vi "NI-USB-8451 SPI EEPROM Programmer.vi"() -> ()   [LabVIEW 2015]
doc: "This example shows a more generalized way to use the SPI advanced API to write data. It allows the user to change the following parameters: page size, write delay, the endianness of the address bytes, and the number of bytes in an address.\n\nThe parameters will have the following effects:\n\nTarget Page Size (bytes): This places an additional constraint on the amount of bytes written. The smaller value will be used, and that number of bytes written.\nWrite Delay Between Pages (ms): This will force a mandatory delay after writing bytes to a device.\nData Address Width: This will allow the user to specify the EEPROM Data Address as either 1 or 2 bytes.\nData Address Endianness: This control will change the ordering of the bytes in the EEPROM Data Address, note that this only has an effect if there are 2 bytes in the address.\n\nFor connection information see the NI-845x Hardware and Software manual and the manual for your specific SPI device."
uses:
  <vilib>/ni845x/ni845x.llb/ni845xControl.ctl
  <vilib>/ni845x/ni845x.llb/ni845xSpiScriptControl.ctl
  <vilib>/ni845x/ni845x.llb/NI-845x SPI Script Us Delay.vi
  <vilib>/ni845x/ni845x.llb/NI-845x SPI Script Ms Delay.vi
  <vilib>/ni845x/ni845x.llb/NI-845x SPI Close Script Reference.vi
  <vilib>/LAVA/UI Tools/Dialog/Dialog/Dialog/Dialog__lava_lib_ui_tools.lvclass
  <resource>/objmgr/NI845x.rc
panel:
  in  "Verbose?":bool
  in  "Tab Control":T1(tab)
  in  "EEPROM Program Data":string[][](table)
  out "Data Bytes Written":u8[](array[numeric]) format="%x"
  out "Read Data":u8[](array[numeric]) format="%x"
  out "Hex Table":string[][](table)
  out "Bin Table":string[][](table)
  in  "EEPROM Device Type":enum16{"Microchip 93C86", "Microchip LC56BT"}(ring)=enum."Microchip LC56BT"
  in  "Device Mode":enum16{"SPI", "I2C", "DIO"}(ring)
  in  "CS Idle Level":enum16{"Low (Assert High)", "High (Assert Low)"}(ring)
  in  "CLK Phase (CPHS)":i32(ring) items=["0 (First Edge)", "1 (Second Edge)"]
  in  "CLK Polarity (CPOL)":i32(ring) items=["0 (Idle Low)", "1 (Idle High)"]
  in  "IO Level (V)":i32(ring)=33 items=["3.3V"=33, "2.5V"=25, "1.8V"=18, "1.5V"=15, "1.2V"=12]
  in  "CS/SS":u32
  in  "NI8451 Device ID":T2="NI-8451"
  in  "CLK Rate (kHz)":u16=2000
  in  "Config INI Save":bool
  in  "Help":bool
  in  "QUIT":bool
  in  "Data Width":enum16{"8 bits", "16 bits"}(ring)
  in  "Address Width":enum16{"8 bits", "16 bits"}(ring)
  in  "Bit Pattern (Write All)":T3(ring)=enum."All ONES"
  in  "Data Address Endianness":bool=TRUE
  in  "Page Write Delay (ms)":u8=3
  in  "Target Page Size (bytes)":i32=2 min=2 max=65535 step=2 format="%04x"
  in  "EEPROM Address (u8)":u16 format="%04x"
  in  "Number of Bytes (Read)":i16=256 min=4 step=4 format="%04x"
  in  "WRAL":u8=17 format="%08b"
  in  "ERAL":u8=18 format="%08b"
  in  "EWEN":u8=19 format="%08b"
  in  "READ":u8=6 format="%08b"
  in  "WRITE":u8=5 format="%08b"
  in  "EWDS":u8=16 format="%08b"
  in  "Write ALL Device":bool
  in  "Erase ALL Device":bool
  in  "Read Device":bool
  in  "Program Device":bool
  in  "SPI Script Reference":T4
  # "NI-USB-8451 SPI/I2C EEPROM Programmer\n(for 8-bit Devices Only)"
  # "NI-8451 Device Configuration"
  # "Slave Device Configur ation"
  # "Big Endian"
  # "Little Endian"
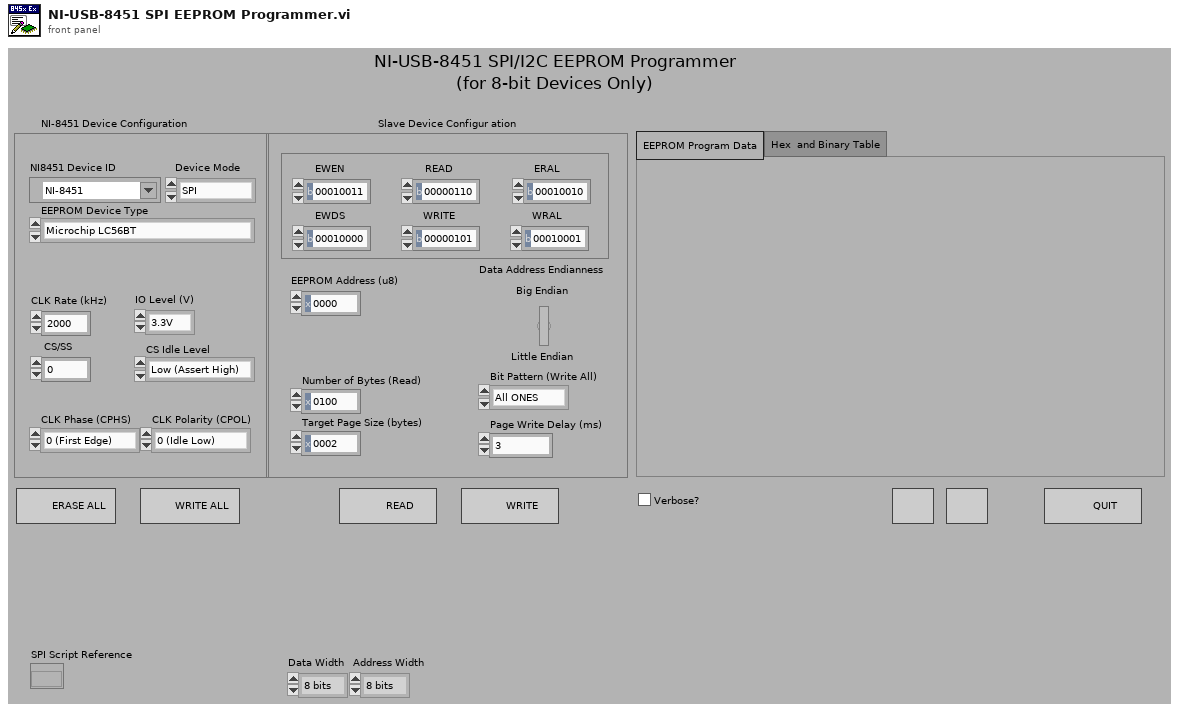
[diagram p1: front panel]
types:
  T1 = enum32{"EEPROM Program Data", "Hex  and Binary Table"}
  T2 = typedef "ni845xControl.ctl" = refnum<k21>
  T3 = enum8{"0xEE (0b11101110)", "0xAA (0b10101010)", "0x55 (0b01010101)", "All ONES", "All ZEROES", ""}
  T4 = typedef "ni845xSpiScriptControl.ctl" = refnum<k20>
  T5 = enum32{"Invalid", "Standard", "Closed", "Hidden", "Minimized", "Maximized"}
  T6 = enum32{"invalid app kind", "Development System", "Run Time System", "Student Edition", "Embedded LabVIEW", "Evaluation", "Custom"}
  T7 = cluster{"INI Path":path, "SPI Script Reference":T4, "NI8451 Device ID":T2, "Device Mode":enum16{"SPI", "I2C", "DIO"}, "EEPROM Device Type":enum16{"Microchip 93C86", "Microchip LC56BT"}, "Core":cluster{"Current VI Reference":refnum<vi>, "Close Panel on Exit?":bool}, "IO Level (V)":i32, "CS/SS":u32, "CLK Rate (kHz)":u16, "CLK Polarity (CPOL)":i32, "CLK Phase (CPHS)":i32, " Address Width":enum16{"8 bits", "16 bits"}, "Data Width":enum16{"8 bits", "16 bits"}, "EEPROM Address (u8)":u16, "Number of Bytes (Read)":i16, "Target Page Size (bytes)":i32, "Page Write Delay (ms)":u8, "Array of Write Cluster Information":cluster{"EEPROM Address":u16, "Length":u32, "Data Index":u32}[], "CS Idle Level":enum16{"Low (Assert High)", "High (Assert Low)"}, "script read index":u32, "Bit Pattern (Write All)":enum8{"0xEE (0b11101110)", "0xAA (0b10101010)", "0x55 (0b01010101)", "All ONES", "All ZEROES", ""}, "READ":u8, "WRITE":u8, "EWEN":u8, "EWDS":u8, "WRAL":u8, "ERAL":u8, "Hex Table":string[][], "Bin Table ":string[][], "EEPROM Program Data ":string[][], "Read Data":u8[], "Data Bytes Written":u8[], "Data Address Endianness":bool, "Verbose?":bool}
  T8 = cluster{"Current VI Reference":refnum<vi>, "Close Panel on Exit?":bool}
  T9 = cluster{"EEPROM Address":u16, "Length":u32, "Data Index":u32}[]
  T10 = typedef "imagedata.ctl" = cluster{"image type":i32, "image depth":i32, "image":u8[], "mask":u8[], "colors":u32[], "Rectangle":cluster{"left":i16, "top":i16, "right":i16, "bottom":i16}}
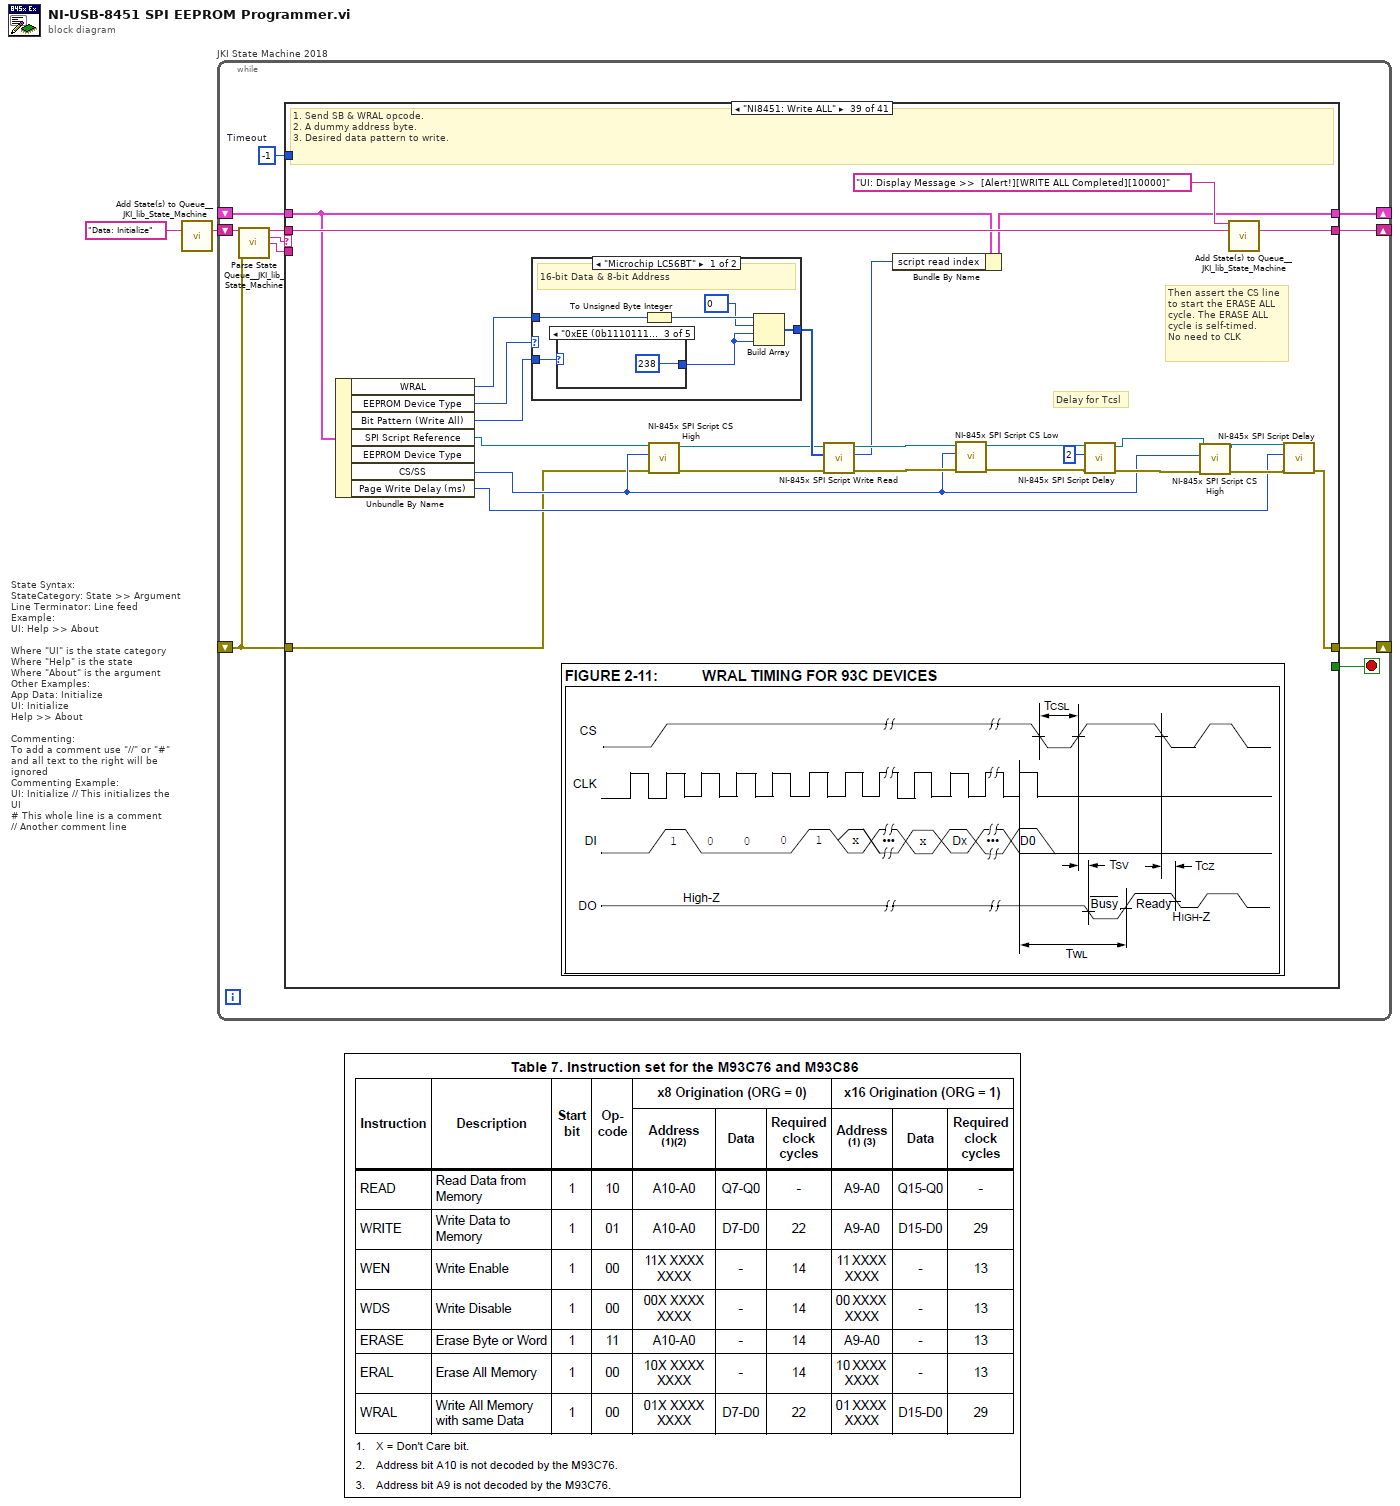
[diagram p0: block diagram]
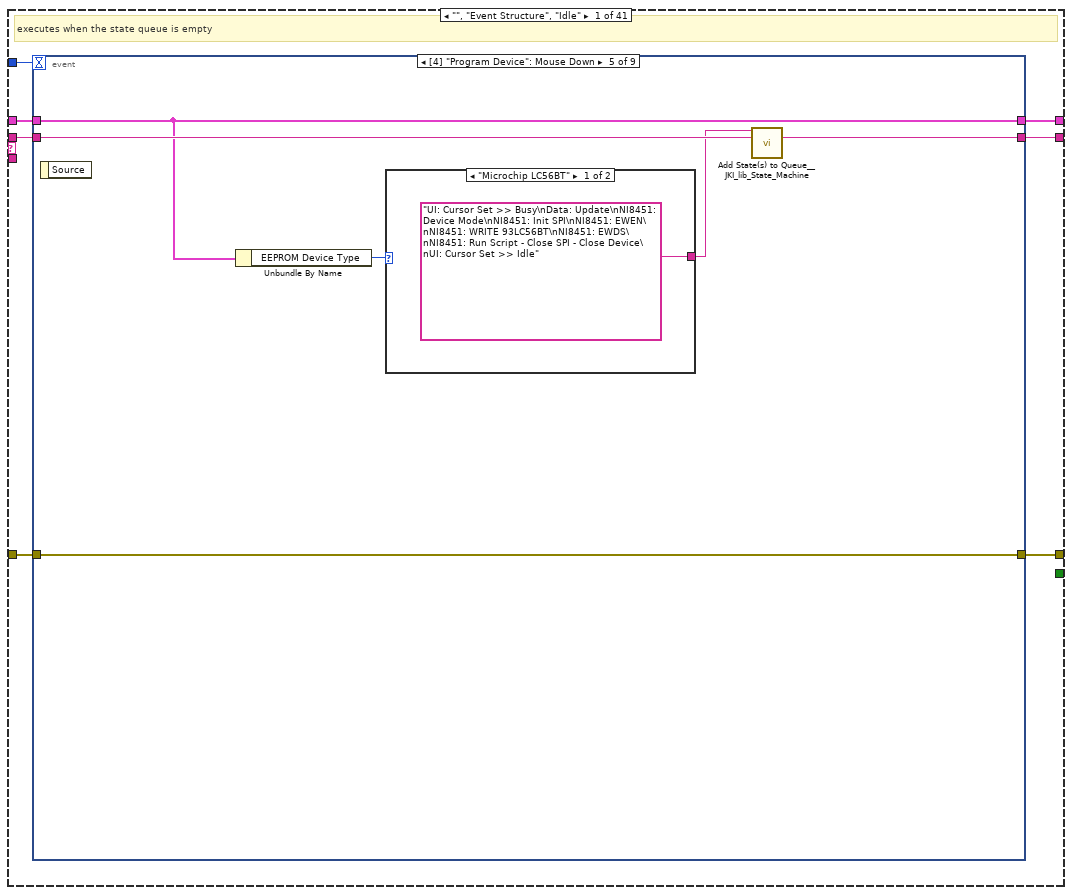
[diagram p2: hidden frame]
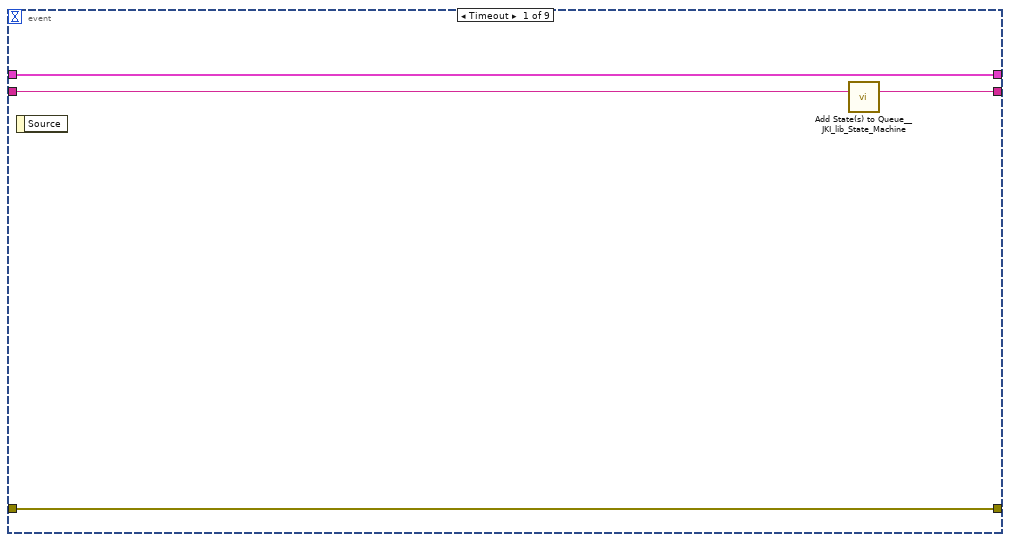
[diagram p3: hidden frame]
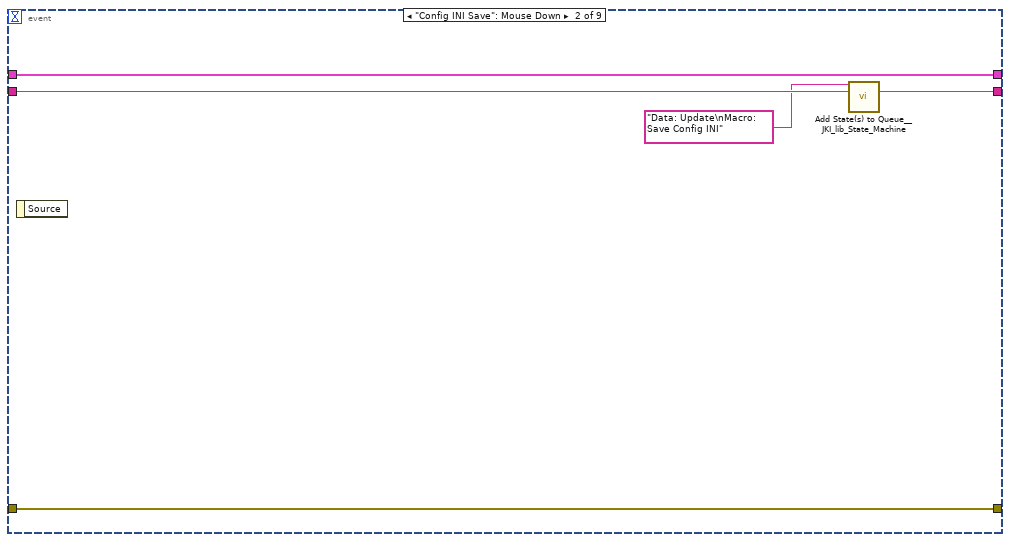
[diagram p4: hidden frame]
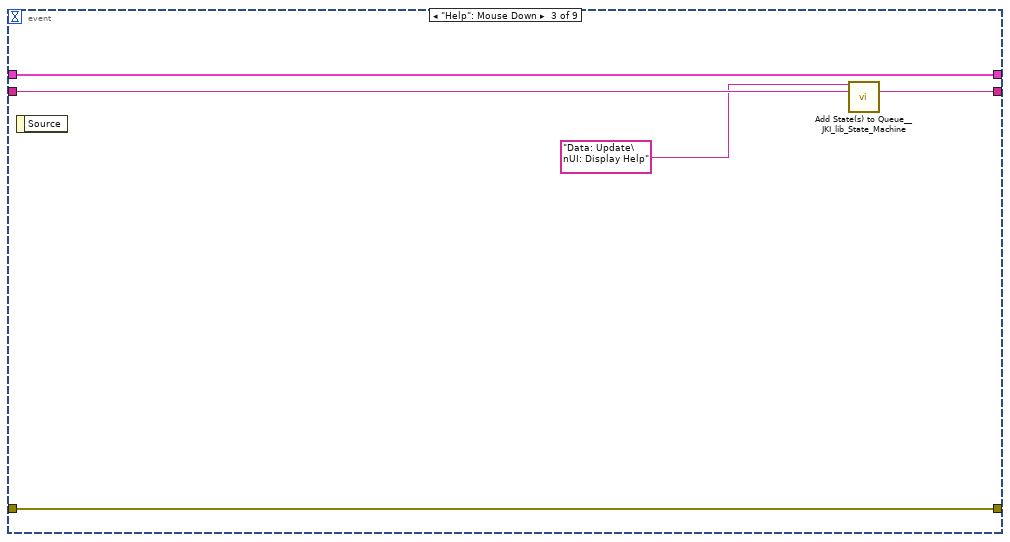
[diagram p5: hidden frame]
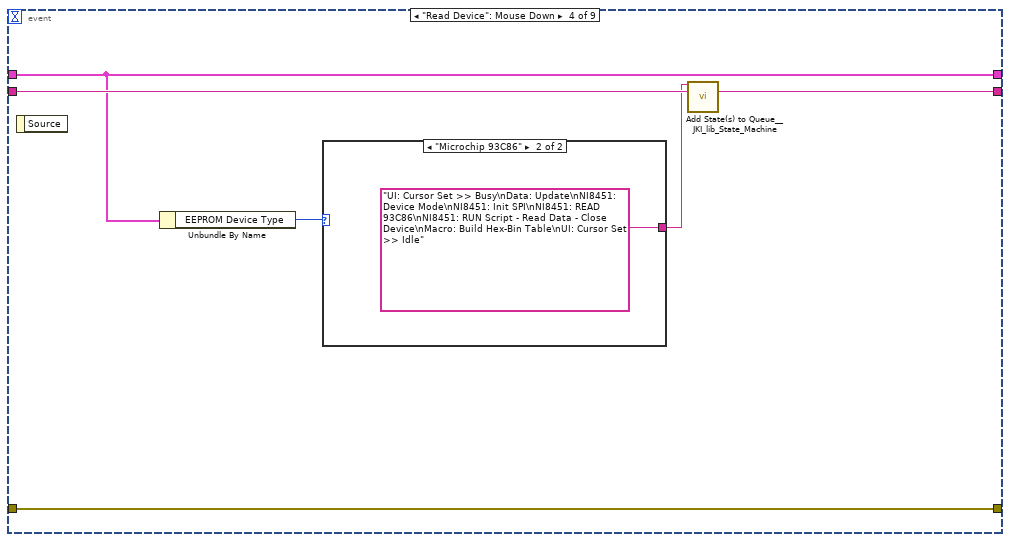
[diagram p6: hidden frame]
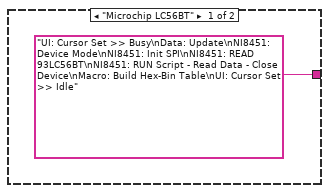
[diagram p7: hidden frame]
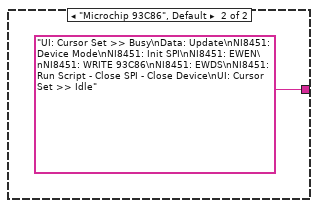
[diagram p8: hidden frame]
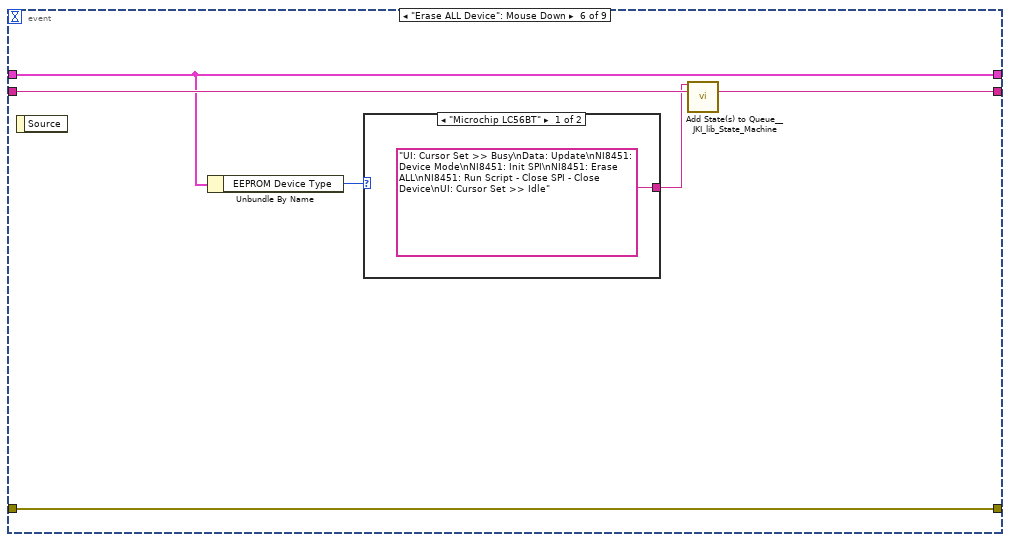
[diagram p9: hidden frame]
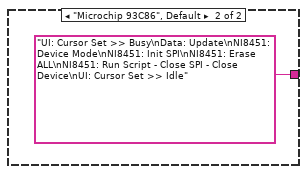
[diagram p10: hidden frame]
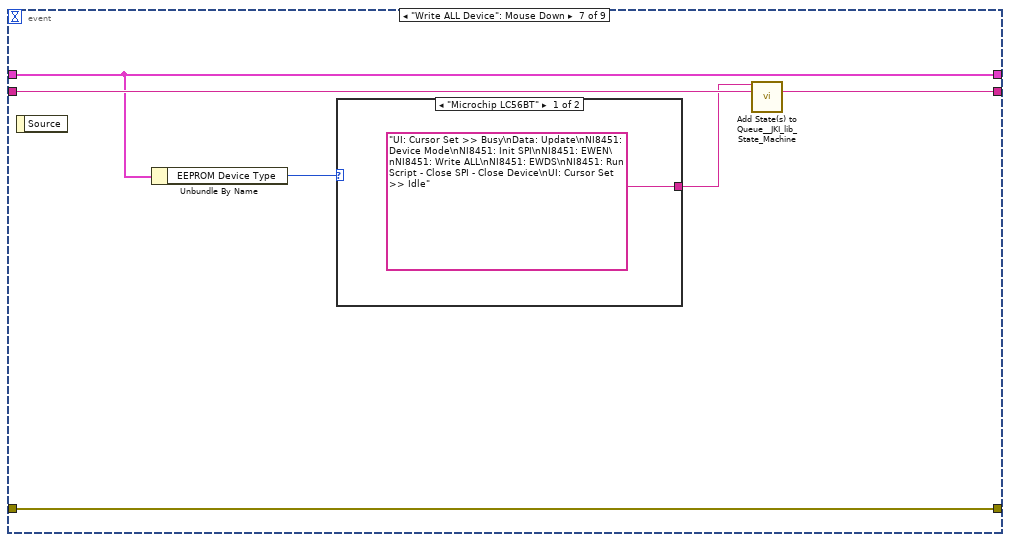
[diagram p11: hidden frame]
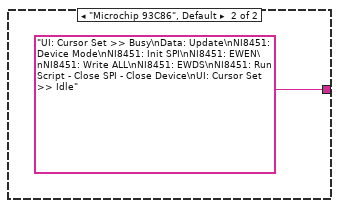
[diagram p12: hidden frame]
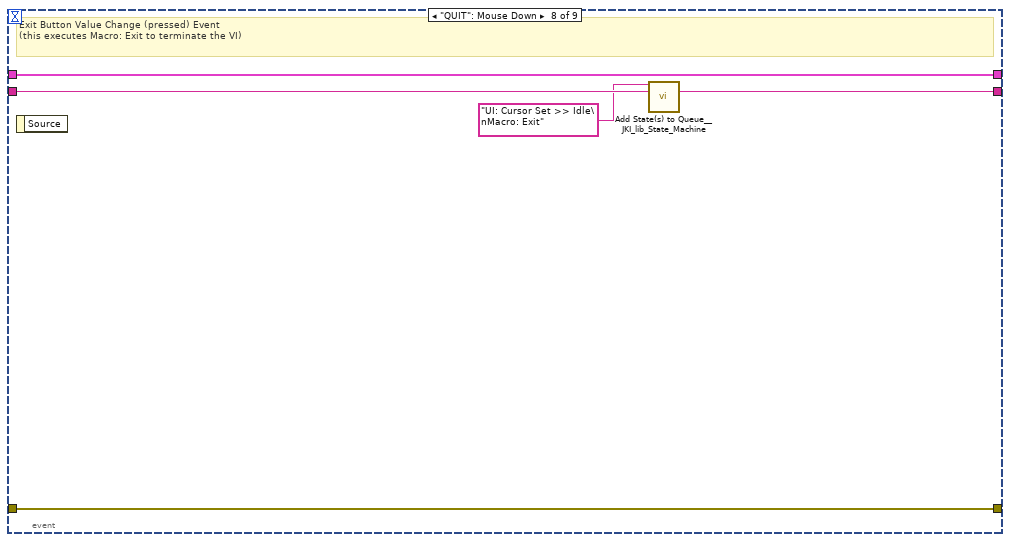
[diagram p13: hidden frame]
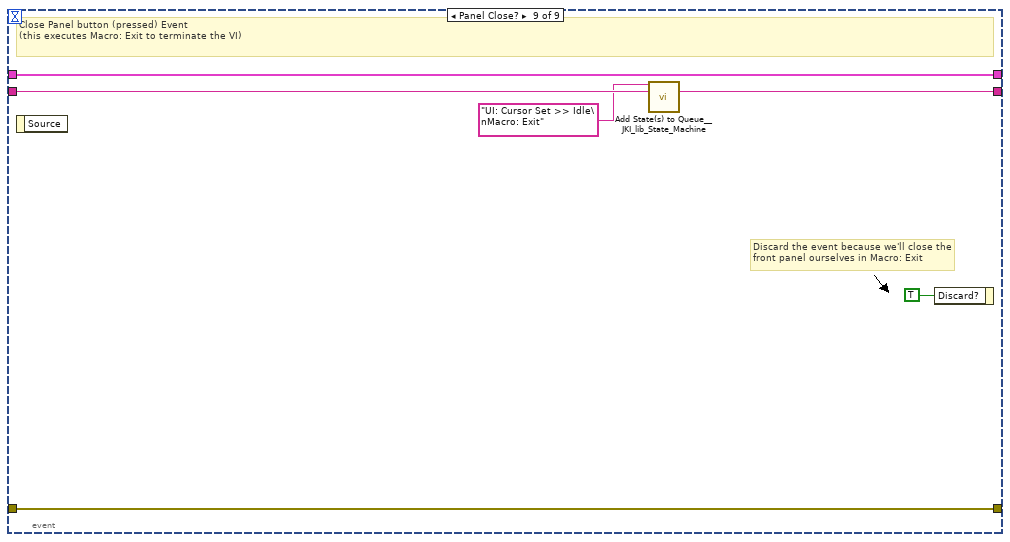
[diagram p14: hidden frame]
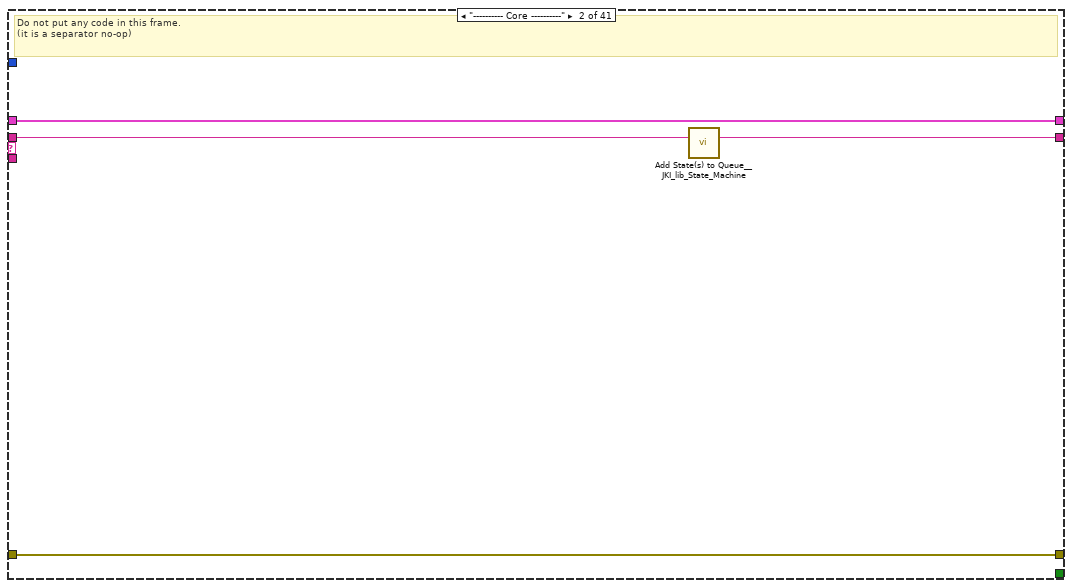
[diagram p15: hidden frame]
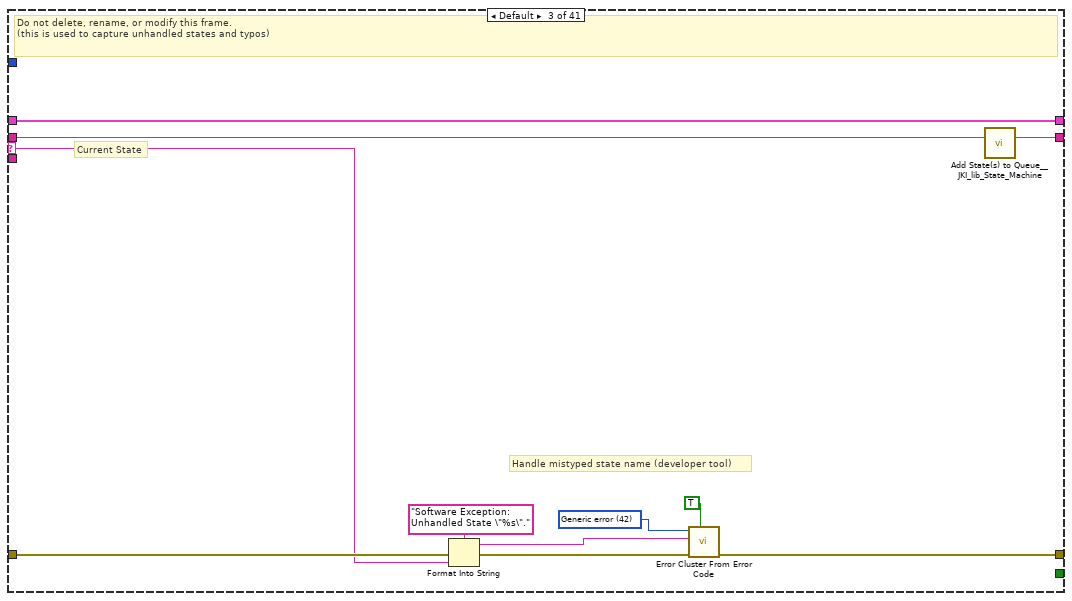
[diagram p16: hidden frame]
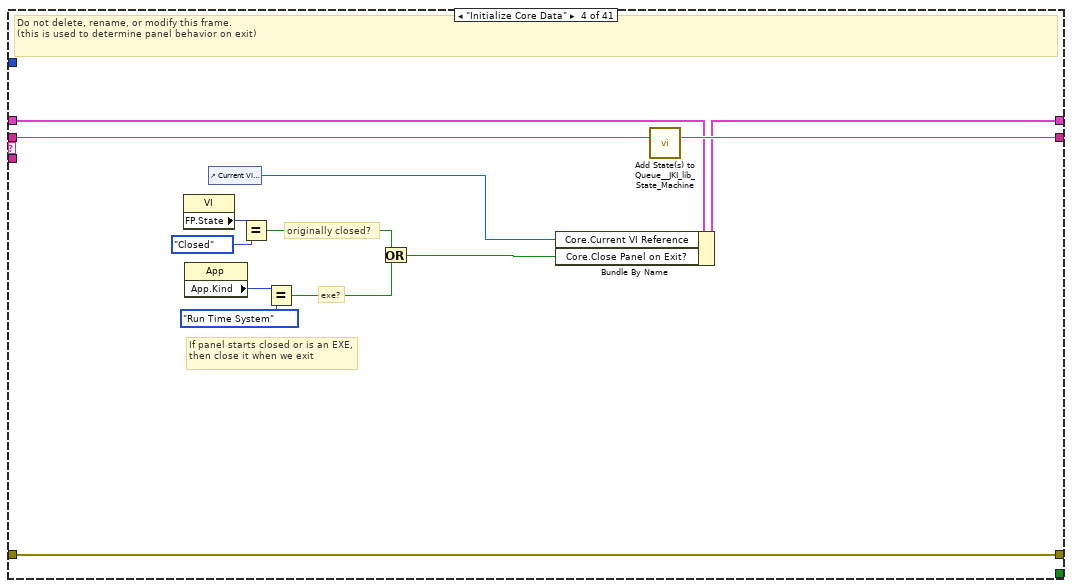
[diagram p17: hidden frame]
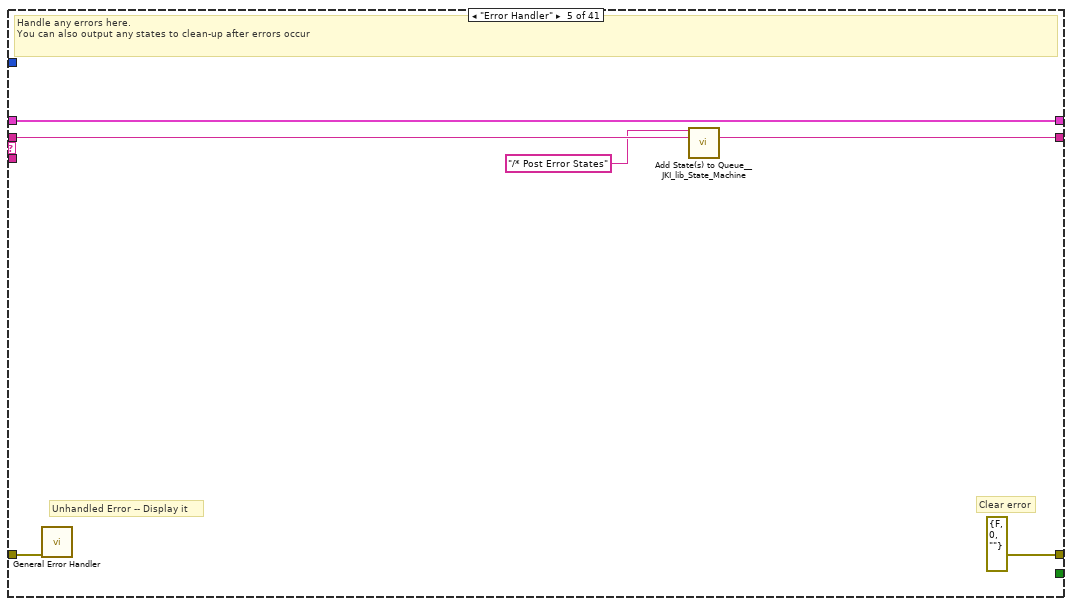
[diagram p18: hidden frame]
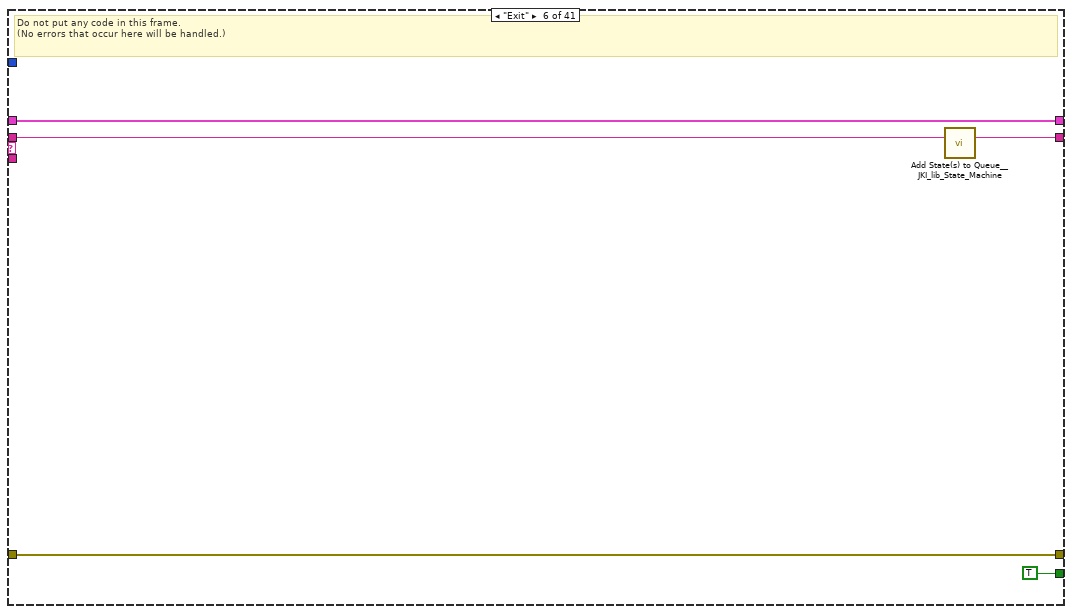
[diagram p19: hidden frame]
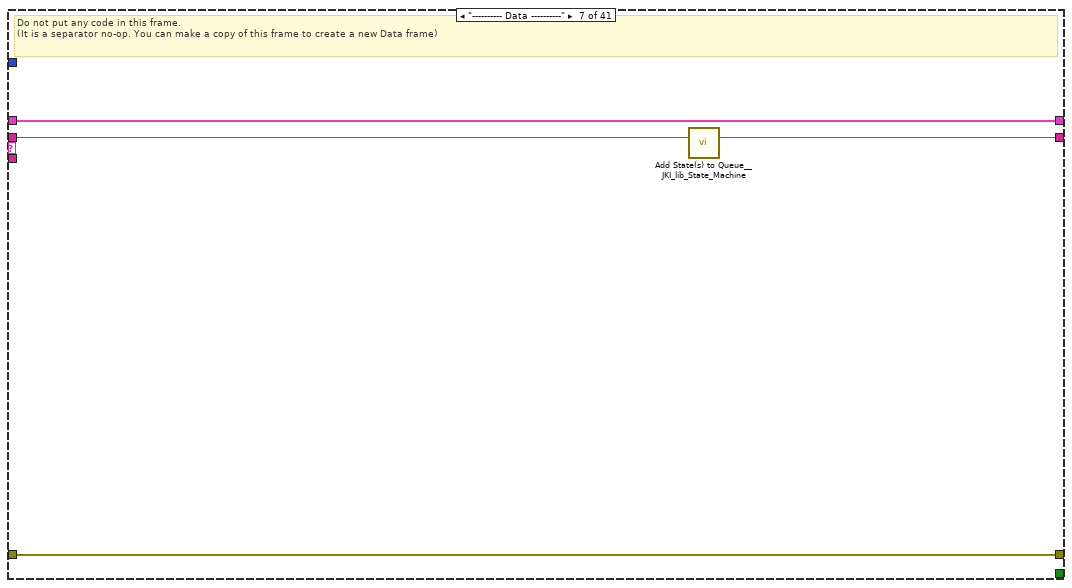
[diagram p20: hidden frame]
diagram:
  # "State Syntax:\nStateCategory: State >> Argument\nLine Terminator: Line feed\nExample:\nUI: Help >> About\n\nWhere \"UI\" is the state category\nWhere \"Help\" is the state\nWhere \"About\" is the argument\nOther Examples:\nApp Data: Initialize\nUI: Initialize\nHelp >> About\n\nCommenting:\nTo add a comment use \"//\" or \"#\" and all text to the right will be ignored\nCommenting Example:\nUI: Initialize // This initializes the UI\n# This whole line is a comment\n// Another comment line"
  n1 = call <vilib>:"Add State(s) to Queue__JKI_lib_State_Machine.vi"("State(s) in (\"\")"="Data: Initialize") -> ("States Out"=w2:string)  [unwired: 14 in]
  n2 = while "JKI State Machine 2018" {
    shift-right: [w6] -> _
    shift-left: _ -> [w5]
    shift-right: [w9] -> _
    shift-left: _ -> [w3]
    shift-right: [w8] -> _
    shift-left: w2 -> [w10]
    stop <- w7 stop-if-true
    w4 = -1  # Timeout
    n3 = call <vilib>:"Parse State Queue__JKI_lib_State_Machine.vi"("State Queue"=w10, "Error In (no error)"=w3) -> ("Remaining States"=w12:string, "Current State"=w13:string, "Arguments"=w11:string)  [unwired: 11 in]
    n4 = case shown="\"NI8451: Write ALL\"" w13 {
      selector: w13 -> [_ _ w82 _ _ _ _ _ _ _ _ _ _ _ _ _ _ _ _ _ _ _ _ _ _ _ _ _ _ _ _ _ _ _ _ _ _ _ _ _ _]
      tunnel: w12 -> [w20 w81 w86 w105 w111 w116 w120 w165 w190 w196 w200 w204 w210 w221 w296 w304 w341 w359 w369 w383 w431 w443 w455 w459 w463 w466 w470 w472 w501 w526 w577 w610 w677 w735 w805 w889 w985 w1039 w1103 w1143 w1156]
      tunnel: w11 -> [_ _ _ _ _ _ _ _ _ _ _ _ w205 w215 _ w300 _ _ _ _ _ _ _ _ _ _ _ _ _ _ _ _ _ _ _ _ _ _ _ _ _]
      tunnel: w5 -> [w18 w78 w84 w98 w108 w114 w117 _ w169 w191 w197 w202 w208 w217 w294 w298 w338 w357 w366 w380 w424 w437 w446 w456 w460 w464 w467 w474 w491 w517 w569 w607 w671 w732 w801 w886 w978 w1033 w1098 w1136 w1149]
      tunnel: [w17 w79 w88 w102 errorcluster {"status"=FALSE, "code"=0, "source"=""} ("error out") w113 w118 w130 w188 w192 w198 w201 w206 w218 w293 w302 w339 w349 w367 w381 w420 w440 w449 w457 w461 w465 w468 w475 w481 w518 w557 w601 w661 w726 w799 w879 w979 w1015 w1082 w1138 w1151] -> w9
      tunnel: w3 -> [w16 w79 w87 w102 w107 w113 w118 w125 w188 w193 w198 w201 w207 w219 w291 w301 w339 w348 w367 w381 w429 w441 w450 w457 w461 w465 w468 w475 w485 w519 w568 w608 w657 w733 w800 w887 w975 w1034 w1079 w1139 w1152]
      tunnel: [w19 w80 w85 w104 w110 w115 w119 w164 w189 w195 w199 w203 w209 w220 w295 w303 w340 w358 w368 w382 w430 w442 w454 w458 w462 w466 w469 w476 w500 w525 w576 w609 w676 w734 w804 w888 w984 w1038 w1102 w1142 w1155] -> w8
      tunnel: [_ _ _ _ _ TRUE _ _ _ _ _ _ _ _ _ _ _ _ _ _ _ _ _ _ _ _ _ _ _ _ _ _ _ _ _ _ _ _ _ _ _] -> w7
      tunnel: [w15 w78 w84 w103 w108 w114 w117 w137 w187 w191 w197 w202 w208 w217 w294 w298 w338 w357 w366 w375 w424 w437 w446 w456 w460 w464 w467 w474 w480 w517 w565 w605 w668 w730 w795 w882 w978 w1019 w1086 w1126 w1149] -> w6
      tunnel: w4 -> [w14 _ _ _ _ _ _ _ _ _ _ _ _ _ _ _ _ _ _ _ _ _ _ _ _ _ _ _ _ _ _ _ _ _ _ _ _ _ _ _ _]
      frame "", "Event Structure", "Idle" {
        # "executes when the state queue is empty"
        n5 = event shown="[4] \"Program Device\": Mouse Down" {
          selector: _ -> [_ _ _ _ _ _ _ _ _]
          dyn-events: _ -> [_ _ _ _ _ _ _ _ _]
          timeout: w14 -> [_ _ _ _ _ _ _ _ _]
          tunnel: w20 -> [w24 w29 w34 w39 w47 w55 w63 w71 w77]
          tunnel: [w23 w28 w33 w38 w46 w54 w62 w70 w76] -> w19
          tunnel: w18 -> [w21 w26 w31 w36 w44 w52 w60 w68 w74]
          tunnel: [w22 w27 w32 w40 w48 w56 w64 w69 w75] -> w17
          tunnel: w16 -> [w22 w27 w32 w40 w48 w56 w64 w69 w75]
          tunnel: [w21 w26 w31 w36 w44 w52 w60 w68 w74] -> w15
          event Timeout {
            n6 = event-data() -> ()  [unwired: 1 in, 1 out]
            n7 = call <vilib>:"Add State(s) to Queue__JKI_lib_State_Machine.vi"("State(s) in (\"\")"=w24) -> ("States Out"=w23:string)  [unwired: 14 in]
          }
          event "Config INI Save": Mouse Down {
            n8 = event-data() -> ()  [unwired: 1 in, 1 out]
            n9 = call <vilib>:"Add State(s) to Queue__JKI_lib_State_Machine.vi"("State(s) in Front (\"\")"="Data: Update\nMacro: Save Config INI" ("State(s) in Front (\"\")"), "State(s) in (\"\")"=w29) -> ("States Out"=w28:string)  [unwired: 13 in]
          }
          event "Help": Mouse Down {
            n10 = event-data() -> ()  [unwired: 1 in, 1 out]
            n11 = call <vilib>:"Add State(s) to Queue__JKI_lib_State_Machine.vi"("State(s) in Front (\"\")"="Data: Update\nUI: Display Help" ("State(s) in Front (\"\")"), "State(s) in (\"\")"=w34) -> ("States Out"=w33:string)  [unwired: 13 in]
          }
          event "Read Device": Mouse Down {
            n12 = event-data() -> ()  [unwired: 1 in, 1 out]
            n13 = Unbundle By Name(w36) -> ("EEPROM Device Type"=w35:enum16{"Microchip 93C86", "Microchip LC56BT"})
            n14 = case shown="\"Microchip 93C86\"" w35 {
              tunnel: ["UI: Cursor Set >> Busy\nData: Update\nNI8451: Device Mode\nNI8451: Init SPI\nNI8451: READ 93LC56BT\nNI8451: RUN Script - Read Data - Close Device\nMacro: Build Hex-Bin Table\nUI: Cursor Set >> Idle" ("State(s) in Front (\"\")") "UI: Cursor Set >> Busy\nData: Update\nNI8451: Device Mode\nNI8451: Init SPI\nNI8451: READ 93C86\nNI8451: RUN Script - Read Data - Close Device\nMacro: Build Hex-Bin Table\nUI: Cursor Set >> Idle" ("State(s) in Front (\"\")")] -> w37
              frame "Microchip LC56BT" {
              }
              frame "Microchip 93C86" {
              }
            }
            n15 = call <vilib>:"Add State(s) to Queue__JKI_lib_State_Machine.vi"("State(s) in Front (\"\")"=w37, "State(s) in (\"\")"=w39) -> ("States Out"=w38:string)  [unwired: 13 in]
          }
          event "Program Device": Mouse Down {
            n16 = event-data() -> ()  [unwired: 1 in, 1 out]
            n17 = Unbundle By Name(w44) -> ("EEPROM Device Type"=w43:enum16{"Microchip 93C86", "Microchip LC56BT"})
            n18 = case shown="\"Microchip LC56BT\"" w43 {
              tunnel: ["UI: Cursor Set >> Busy\nData: Update\nNI8451: Device Mode\nNI8451: Init SPI\nNI8451: EWEN\nNI8451: WRITE 93LC56BT\nNI8451: EWDS\nNI8451: Run Script - Close SPI - Close Device\nUI: Cursor Set >> Idle" ("State(s) in Front (\"\")") "UI: Cursor Set >> Busy\nData: Update\nNI8451: Device Mode\nNI8451: Init SPI\nNI8451: EWEN\nNI8451: WRITE 93C86\nNI8451: EWDS\nNI8451: Run Script - Close SPI - Close Device\nUI: Cursor Set >> Idle" ("State(s) in Front (\"\")")] -> w45
              frame "Microchip LC56BT" {
              }
              frame "Microchip 93C86", Default {
              }
            }
            n19 = call <vilib>:"Add State(s) to Queue__JKI_lib_State_Machine.vi"("State(s) in Front (\"\")"=w45, "State(s) in (\"\")"=w47) -> ("States Out"=w46:string)  [unwired: 13 in]
          }
          event "Erase ALL Device": Mouse Down {
            n20 = event-data() -> ()  [unwired: 1 in, 1 out]
            n21 = Unbundle By Name(w52) -> ("EEPROM Device Type"=w51:enum16{"Microchip 93C86", "Microchip LC56BT"})
            n22 = case shown="\"Microchip LC56BT\"" w51 {
              tunnel: ["UI: Cursor Set >> Busy\nData: Update\nNI8451: Device Mode\nNI8451: Init SPI\nNI8451: Erase ALL\nNI8451: Run Script - Close SPI - Close Device\nUI: Cursor Set >> Idle" ("State(s) in Front (\"\")") "UI: Cursor Set >> Busy\nData: Update\nNI8451: Device Mode\nNI8451: Init SPI\nNI8451: Erase ALL\nNI8451: Run Script - Close SPI - Close Device\nUI: Cursor Set >> Idle" ("State(s) in Front (\"\")")] -> w53
              frame "Microchip LC56BT" {
              }
              frame "Microchip 93C86", Default {
              }
            }
            n23 = call <vilib>:"Add State(s) to Queue__JKI_lib_State_Machine.vi"("State(s) in Front (\"\")"=w53, "State(s) in (\"\")"=w55) -> ("States Out"=w54:string)  [unwired: 13 in]
          }
          event "Write ALL Device": Mouse Down {
            n24 = event-data() -> ()  [unwired: 1 in, 1 out]
            n25 = Unbundle By Name(w60) -> ("EEPROM Device Type"=w59:enum16{"Microchip 93C86", "Microchip LC56BT"})
            n26 = case shown="\"Microchip LC56BT\"" w59 {
              tunnel: ["UI: Cursor Set >> Busy\nData: Update\nNI8451: Device Mode\nNI8451: Init SPI\nNI8451: EWEN\nNI8451: Write ALL\nNI8451: EWDS\nNI8451: Run Script - Close SPI - Close Device\nUI: Cursor Set >> Idle" ("State(s) in Front (\"\")") "UI: Cursor Set >> Busy\nData: Update\nNI8451: Device Mode\nNI8451: Init SPI\nNI8451: EWEN\nNI8451: Write ALL\nNI8451: EWDS\nNI8451: Run Script - Close SPI - Close Device\nUI: Cursor Set >> Idle" ("State(s) in Front (\"\")")] -> w61
              frame "Microchip LC56BT" {
              }
              frame "Microchip 93C86", Default {
              }
            }
            n27 = call <vilib>:"Add State(s) to Queue__JKI_lib_State_Machine.vi"("State(s) in Front (\"\")"=w61, "State(s) in (\"\")"=w63) -> ("States Out"=w62:string)  [unwired: 13 in]
          }
          event "QUIT": Mouse Down {
            # "Exit Button Value Change (pressed) Event\n(this executes Macro: Exit to terminate the VI)"
            n28 = event-data() -> ()  [unwired: 1 in, 1 out]
            n29 = call <vilib>:"Add State(s) to Queue__JKI_lib_State_Machine.vi"("State(s) in Front (\"\")"="UI: Cursor Set >> Idle\nMacro: Exit", "State(s) in (\"\")"=w71) -> ("States Out"=w70:string)  [unwired: 13 in]
          }
          event Panel Close? {
            # "Discard the event because we'll close the front panel ourselves in Macro: Exit"
            # "Close Panel button (pressed) Event\n(this executes Macro: Exit to terminate the VI)"
            n30 = event-data() -> ()  [unwired: 1 in, 1 out]
            n31 = call <vilib>:"Add State(s) to Queue__JKI_lib_State_Machine.vi"("State(s) in Front (\"\")"="UI: Cursor Set >> Idle\nMacro: Exit", "State(s) in (\"\")"=w77) -> ("States Out"=w76:string)  [unwired: 13 in]
            n32 = event-data("Discard?"=TRUE) -> ()  [unwired: 1 in, 1 out]
          }
        }
      }
      frame "---------- Core ----------" {
        # "Do not put any code in this frame.\n(it is a separator no-op)"
        n33 = call <vilib>:"Add State(s) to Queue__JKI_lib_State_Machine.vi"("State(s) in (\"\")"=w81) -> ("States Out"=w80:string)  [unwired: 14 in]
      }
      frame Default {
        w91 = 42 items=["No error", "Argument error", "Memory is full", "Out of zone", "End of file", "File already open", "Generic file I/O error", "File not found", "File permission error", "Disk is full", "Duplicate path", "Too many files open", "System feature not enabled", "Resource file not found", "Cannot add resource", "Resource not found", "Image not found", "Image memory error", "Pen does not exist", "Config type invalid", "Config token not found", "Config parse error", "Config memory error", "Bad external code format", "Bad external code offset", "External code not present", "Null window", "Destroy window error", "Null menu", "Print aborted", "Bad print record", "Print driver error", "Windows error during printing", "Memory error during printing", "Print dialog error", "Generic print error", "Invalid device refnum", "Device not found", "Device parameter error", "Device unit error", "Cannot open device", "Device call aborted", "Generic error", "Cancelled by user", "Object ID too low", "Object ID too high", "Object not in heap", "Unknown heap", "Unknown object (invalid DefProc)", "Unknown object (DefProc not in table)", "Message out of range", "Invalid (null) method", "Unknown message", "Manager call not supported", "Bad address", "Network operation in progress", "Network operation timed out", "Connection is busy", "Network attribute not supported", "Network error", "Address in use", "System out of memory", "Connection aborted", "Connection refused", "Not connected", "Already connected", "Connection closed", "Initialization error (interapplication manager)", "Bad occurrence", "Wait on unbound occurrence handler", "Occurrence queue overflow", "Datalog type conflict", "Unused", "Unrecognized type (interapplication manager)", "Memory corrupt", "Failed to make temporary DLL", "Old CIN version", "Drag socket not found", "Failed to load drop-object", "Failed to register OLE object", "Failed to release OLE object", "Format specifier type mismatch", "Unknown format specifier", "Too few format specifiers", "Too many format specifiers", "Scan failed", "Newer CIN version", "Error converting to variant", "Runtime menu error", "Password tampered", "Variant attribute not found", "Incompatible variant data type", "Event data is not available", "Event Store is not present", "Occurrence is not found", "Event Queue is not created", "Event info is not available", "Refnum passed is NULL", "Error retrieving Class GUID", "Error retrieving CoClass GUID", "Error retrieving TypeLib GUID.", "Bad built application magic bytes.", "Specific driver is different from the specific driver associated with the Logical Name.", "There is no session opened to the class driver.", "Max Error", "MAX - Error with config objects", "MAX - Error loading configuration", "MAX - Group not supported"]
        # "Current State"
        # "Handle mistyped state name (developer tool)"
        # "Do not delete, rename, or modify this frame.\n(this is used to capture unhandled states and typos)"
        n34 = Format Into String(format string="Software Exception: Unhandled State \"%s\"." ("message"), error in=w87, w82) -> (resulting string=w90:string, error out=w89:errorcluster)  [unwired: 1 in]
        n35 = call <vilib>:"Error Cluster From Error Code.vi"("show call chain? (False)"=TRUE, "error in (no error)"=w89, "error message (\"\")"=w90, "error code (0)"=w91) -> ("error out"=w88:errorcluster)  [unwired: 5 in]
        n36 = call <vilib>:"Add State(s) to Queue__JKI_lib_State_Machine.vi"("State(s) in (\"\")"=w86) -> ("States Out"=w85:string)  [unwired: 14 in]
      }
      frame "Initialize Core Data" {
        # "originally closed?"
        # "exe?"
        # "If panel starts closed or is an EXE, then close it when we exit"
        # "Do not delete, rename, or modify this frame.\n(this is used to determine panel behavior on exit)"
        n37 = property class="VI"() -> ("FP.State"=w95:T5)  [unwired: 2 in, 2 out]
        n38 = property class="App"() -> ("App.Kind"=w101:T6)  [unwired: 2 in, 2 out]
        n39 = control-ref of="Current VI Reference"() -> (w96:refnum<vi>)
        n40 = Equal?(x=w95, y=T5."Closed" ("Front Panel Window:State")) -> (x = y?=w93:bool)
        n41 = Equal?(x=w101, y=T6."Run Time System" ("Application:Kind")) -> (x = y?=w99:bool)
        n42 = Or(x=w93, y=w99) -> (x .or. y?=w97:bool)
        n43 = Bundle By Name(cluster=w98, "Core.Current VI Reference"=w96, "Core.Close Panel on Exit?"=w97) -> (w103:T7)
        n44 = call <vilib>:"Add State(s) to Queue__JKI_lib_State_Machine.vi"("State(s) in (\"\")"=w105) -> ("States Out"=w104:string)  [unwired: 14 in]
      }
      frame "Error Handler" {
        # "Unhandled Error -- Display it"
        # "Clear error"
        # "Handle any errors here.\nYou can also output any states to clean-up after errors occur"
        n45 = call <vilib>:"General Error Handler.vi"("error in (no error)"=w107) -> ()  [unwired: 10 in, 5 out]
        n46 = call <vilib>:"Add State(s) to Queue__JKI_lib_State_Machine.vi"("State(s) in Front (\"\")"="/* Post Error States", "State(s) in (\"\")"=w111) -> ("States Out"=w110:string)  [unwired: 13 in]
      }
      frame "Exit" {
        # "Do not put any code in this frame.\n(No errors that occur here will be handled.)"
        n47 = call <vilib>:"Add State(s) to Queue__JKI_lib_State_Machine.vi"("State(s) in (\"\")"=w116) -> ("States Out"=w115:string)  [unwired: 14 in]
      }
      frame "---------- Data ----------" {
        # "Do not put any code in this frame.\n(It is a separator no-op. You can make a copy of this frame to create a new Data frame)"
        n48 = call <vilib>:"Add State(s) to Queue__JKI_lib_State_Machine.vi"("State(s) in (\"\")"=w120) -> ("States Out"=w119:string)  [unwired: 14 in]
      }
      frame "Data: Initialize" {
        w121 = string[][] []  # Bin Table
        w122 = string[][] []  # Hex Table
        w124 = string[][] []  # Hex Table
        w127 = u8[] []  # Data Bytes Written
        w128 = u8[] []  # Read Data
        w138 = path ""  # INI Path
        w148 = u8[] [] ("Read Data")
        w153 = u32 0  # script read index
        w133 = T8 {"Current VI Reference"=refnum, "Close Panel on Exit?"=FALSE}  # Core
        # "do not delete - used by framework"
        # "Initialize variables & master cluster here\n(data names are defined by what you wire into the bundle function)"
        n49 = call "CreateWriteCluster.vi"("Page Size in Bytes"="Target Page Size (bytes)", "EEPROM Starting Address"="EEPROM Address (u8)", "Number of Bytes to Write"="Number of Bytes (Read)") -> ("Array of Write Cluster Information"=w141:T9)  [unwired: 1 in]
        n50 = control-ref of="This VI"() -> (w131:refnum<vi>)
        n51 = call "Set Config INI PATH.vi"("error in (no error)"=w125, "reference"=w131) -> ("error out"=w130:errorcluster, "appended path"=w129:path)  [unwired: 2 in]
        n52 = Bundle("INI Path"=w138, "SPI Script Reference"="SPI Script Reference", "NI8451 Device ID"="NI8451 Device ID", "Device Mode"="Device Mode", "EEPROM Device Type"="EEPROM Device Type", "Core"=w133, "IO Level (V)"="IO Level (V)", "CS/SS"="CS/SS", "CLK Rate (kHz)"="CLK Rate (kHz)", "CLK Polarity (CPOL)"="CLK Polarity (CPOL)", "CLK Phase (CPHS)"="CLK Phase (CPHS)", "Address Width"="Address Width", "Data Width"="Data Width", "EEPROM Address (u8)"="EEPROM Address (u8)", "Number of Bytes (Read)"="Number of Bytes (Read)", "Target Page Size (bytes)"="Target Page Size (bytes)", "Page Write Delay (ms)"="Page Write Delay (ms)", "Array of Write Cluster Information"=w141, "CS Idle Level"="CS Idle Level", "script read index"=w153, "Bit Pattern (Write All)"="Bit Pattern (Write All)", "READ"="READ", "WRITE"="WRITE", "EWEN"="EWEN", "EWDS"="EWDS", "WRAL"="WRAL", "ERAL"="ERAL", "Hex Table"=w122, "Bin Table"=w121, "EEPROM Program Data"="EEPROM Program Data", "Read Data"=w128, "Data Bytes Written"=w127, "Data Address Endianness"="Data Address Endianness", "Verbose?"="Verbose?") -> (w163:T7)  [unwired: 1 in]
        n53 = Bundle By Name(cluster=w163, "INI Path"=w129) -> (w137:T7)
        n54 = call <vilib>:"Add State(s) to Queue__JKI_lib_State_Machine.vi"("State(s) in Front (\"\")"="Initialize Core Data\nMacro: Initialize", "State(s) in (\"\")"=w165) -> ("States Out"=w164:string)  [unwired: 13 in]
        "Read Data" <- w148
        "Data Bytes Written" <- w148
        "Hex Table" <- w124
        "Bin Table" <- w124
      }
      frame "Data: Update" {
        # "Update the master cluster for any config changes"
        n55 = Unbundle By Name(w169) -> ("Hex Table"=w168:string[][], "Bin Table"=w167:string[][])
        n56 = local write "Hex Table"(w168) -> ()
        n57 = local write "Bin Table"(w167) -> ()
        n58 = local read "Number of Bytes (Read)"() -> (w182:i16)
        n59 = local read "Data Address Endianness"() -> (w171:bool)
        n60 = local read "Target Page Size (bytes)"() -> (w180:i32)
        n61 = local read "EEPROM Program Data"() -> (w166:string[][])
        n62 = local read "Page Write Delay (ms)"() -> (w186:u8)
        n63 = local read "EEPROM Address (u8)"() -> (w181:u16)
        n64 = local read "EEPROM Device Type"() -> (w172:enum16{"Microchip 93C86", "Microchip LC56BT"})
        n65 = local read "NI8451 Device ID"() -> (w175:T2)
        n66 = local read "Bit Pattern (Write All)"() -> (w179:T3)
        n67 = local read "Address Width"() -> (w184:enum16{"8 bits", "16 bits"})
        n68 = local read "CLK Rate (kHz)"() -> (w178:u16)
        n69 = local read "Device Mode"() -> (w174:enum16{"SPI", "I2C", "DIO"})
        n70 = local read "CS Idle Level"() -> (w185:enum16{"Low (Assert High)", "High (Assert Low)"})
        n71 = local read "IO Level (V)"() -> (w176:i32)
        n72 = local read "Data Width"() -> (w173:enum16{"8 bits", "16 bits"})
        n73 = local read "Verbose?"() -> (w170:bool)
        n74 = local read "CS/SS"() -> (w177:u32)
        n75 = call "CreateWriteCluster.vi"("Page Size in Bytes"=w180, "EEPROM Starting Address"=w181, "Number of Bytes to Write"=w182) -> ("Array of Write Cluster Information"=w183:T9)  [unwired: 1 in]
        n76 = Bundle By Name(cluster=w169, "EEPROM Device Type"=w172, "NI8451 Device ID"=w175, "Device Mode"=w174, "IO Level (V)"=w176, "CS/SS"=w177, "CLK Rate (kHz)"=w178, "Bit Pattern (Write All)"=w179, "Number of Bytes (Read)"=w182, "Target Page Size (bytes)"=w180, "Page Write Delay (ms)"=w186, "CS Idle Level"=w185, "script read index"=w184, "Data Width"=w173, "EEPROM Address (u8)"=w181, "Array of Write Cluster Information"=w183, "Data Address Endianness"=w171, "Verbose?"=w170, "EEPROM Program Data"=w166) -> (w187:T7)
        n77 = call <vilib>:"Add State(s) to Queue__JKI_lib_State_Machine.vi"("State(s) in (\"\")"=w190) -> ("States Out"=w189:string)  [unwired: 14 in]
      }
      frame "Data: Cleanup" {
        # "Cleanup any data and references, here.\n(this is called automatically, by the Macro: Exit)"
        n78 = Unbundle By Name(w191) -> ("Core.Current VI Reference"=w194:refnum<vi>)
        n79 = Close Reference(reference=w194, error in (no error)=w193) -> (error out=w192:errorcluster)
        n80 = call <vilib>:"Add State(s) to Queue__JKI_lib_State_Machine.vi"("State(s) in (\"\")"=w196) -> ("States Out"=w195:string)  [unwired: 14 in]
      }
      frame "---------- UI ----------" {
        # "Do not put any code in this frame.\n(It is a separator no-op. You can make a copy of this frame to create a new UI frame)"
        n81 = call <vilib>:"Add State(s) to Queue__JKI_lib_State_Machine.vi"("State(s) in (\"\")"=w200) -> ("States Out"=w199:string)  [unwired: 14 in]
      }
      frame "UI: Initialize" {
        # "Initialize the User Interface, here.\n(this is called automatically, by the Macro: Init)"
        n82 = call <vilib>:"Add State(s) to Queue__JKI_lib_State_Machine.vi"("State(s) in (\"\")"=w204) -> ("States Out"=w203:string)  [unwired: 14 in]
      }
      frame "UI: Cursor Set" {
        # "Argument"
        # "Set and Unset Cursor Busy.\n(Usage: \"UI: Cursor Set >> Busy|Idle\")"
        n83 = case shown="\"Busy\"" w205 {
          tunnel: w207 -> [w212 w214]
          tunnel: [w211 w213] -> w206
          frame "Idle", Default {
            n84 = call <vilib>:"Unset Busy.vi"("error in (no error)"=w212) -> ("error out"=w211:errorcluster)  [unwired: 10 in]
          }
          frame "Busy" {
            n85 = call <vilib>:"Set Busy.vi"("error in (no error)"=w214) -> ("error out"=w213:errorcluster)  [unwired: 9 in, 1 out]
          }
        }
        n86 = call <vilib>:"Add State(s) to Queue__JKI_lib_State_Machine.vi"("State(s) in (\"\")"=w210) -> ("States Out"=w209:string)  [unwired: 14 in]
      }
      frame "UI: Front Panel State" {
        # "Argument"
        # "Set Front Panel Open or Closed\n(Usage: \"UI: Front Panel State >> Open|Close\")"
        n87 = Unbundle By Name(w217) -> ("Core.Current VI Reference"=w216:refnum<vi>)
        n88 = case shown="\"Minimize\", \"Minimized\"" w215 {
          tunnel: w219 -> [w227 w242 w253 w266 w279]
          tunnel: [w229 w243 w255 w268 w281] -> w218
          tunnel: w216 -> [w228 w240 w254 w267 w280]
          frame "Open", "Standard", Default {
            w222 = T5."Standard" ("State")
            n89 = property class="VI"(reference=w228, error in=w227) -> (reference out=w225:refnum<vi>, error out=w226:errorcluster, "FP.State"=w224:T5)
            n90 = Not Equal?(x=w224, y=w222) -> (x != y?=w223:bool)
            n91 = case shown="True" w223 {
              tunnel: [w233 w235] -> w229
              tunnel: w226 -> [w232 w235]
              tunnel: w225 -> [w231 _]
              tunnel: w222 -> [w230 _]
              frame True {
                n92 = invoke class="VI" method="FP.Open"(reference=w231, error in=w232, "Activate"=TRUE, "State"=w230) -> (error out=w233:errorcluster)  [unwired: 1 in, 4 out]
              }
              frame False {
              }
            }
          }
          frame "Close", "Closed" {
            n93 = property class="VI"(reference=w240, error in=w242) -> (reference out=w239:refnum<vi>, error out=w241:errorcluster, "FP.State"=w237:T5)
            n94 = Not Equal?(x=w237, y=T5."Closed" ("Front Panel Window:State")) -> (x != y?=w236:bool)
            n95 = case shown="True" w236 {
              tunnel: [w244 w247] -> w243
              tunnel: w241 -> [w244 w246]
              tunnel: w239 -> [_ w245]
              frame False {
              }
              frame True {
                n96 = invoke class="VI" method="FP.Close"(reference=w245, error in=w246) -> (error out=w247:errorcluster)  [unwired: 1 in, 2 out]
              }
            }
          }
          frame "Hidden", "Hide" {
            w248 = T5."Hidden" ("State")
            n97 = property class="VI"(reference=w254, error in=w253) -> (reference out=w251:refnum<vi>, error out=w252:errorcluster, "FP.State"=w250:T5)
            n98 = Not Equal?(x=w250, y=w248) -> (x != y?=w249:bool)
            n99 = case shown="True" w249 {
              tunnel: [w259 w260] -> w255
              tunnel: w252 -> [w258 w260]
              tunnel: w251 -> [w257 _]
              tunnel: w248 -> [w256 _]
              frame True {
                n100 = invoke class="VI" method="FP.Open"(reference=w257, error in=w258, "State"=w256) -> (error out=w259:errorcluster)  [unwired: 2 in, 4 out]
              }
              frame False {
              }
            }
          }
          frame "Minimize", "Minimized" {
            w261 = T5."Minimized" ("State")
            n101 = property class="VI"(reference=w267, error in=w266) -> (reference out=w264:refnum<vi>, error out=w265:errorcluster, "FP.State"=w263:T5)
            n102 = Not Equal?(x=w263, y=w261) -> (x != y?=w262:bool)
            n103 = case shown="True" w262 {
              tunnel: [w272 w273] -> w268
              tunnel: w265 -> [w271 w273]
              tunnel: w264 -> [w270 _]
              tunnel: w261 -> [w269 _]
              frame True {
                n104 = invoke class="VI" method="FP.Open"(reference=w270, error in=w271, "State"=w269) -> (error out=w272:errorcluster)  [unwired: 2 in, 4 out]
              }
              frame False {
              }
            }
          }
          frame "Maximize", "Maximized" {
            w274 = T5."Maximized" ("State")
            n105 = property class="VI"(reference=w280, error in=w279) -> (reference out=w277:refnum<vi>, error out=w278:errorcluster, "FP.State"=w276:T5)
            n106 = Not Equal?(x=w276, y=w274) -> (x != y?=w275:bool)
            n107 = case shown="True" w275 {
              tunnel: [w285 w286] -> w281
              tunnel: w278 -> [w284 w286]
              tunnel: w277 -> [w283 _]
              tunnel: w274 -> [w282 _]
              frame True {
                n108 = invoke class="VI" method="FP.Open"(reference=w283, error in=w284, "State"=w282) -> (error out=w285:errorcluster)  [unwired: 2 in, 4 out]
              }
              frame False {
              }
            }
          }
        }
        n109 = call <vilib>:"Add State(s) to Queue__JKI_lib_State_Machine.vi"("State(s) in (\"\")"=w221) -> ("States Out"=w220:string)  [unwired: 14 in]
      }
      frame "UI: Display Help" {
        n110 = call <vilib>:"Read JPEG File.vi"("error in (no error)"=w291, "path to JPEG file"=path "C:/projects/AldrinA_Test_Apps/NI-845x I2C-SPI Programmer GUI/NI8451_J6_wiring.jpg" ("Path")) -> ("error out"=w290:errorcluster, "image data"=w289:T10)  [unwired: 7 in, 1 out]
        n111 = call <vilib>:"Draw Flattened Pixmap.vi"("image data"=w289, "picture"=picture data[5B]) -> ("new picture"=w288:picture)  [unwired: 7 in]
        n112 = call "Picture Prompt.vi"("error in (no error)"=w290, "2D Picture 2"=w288) -> ("error out"=w293:errorcluster)  [unwired: 9 in]
        n113 = call <vilib>:"Add State(s) to Queue__JKI_lib_State_Machine.vi"("State(s) in (\"\")"=w296) -> ("States Out"=w295:string)  [unwired: 14 in]
      }
      frame "UI: Display Message" {
        # "// Command Format:  \"UI: Display Message >> [Window Title] [Message] [Timeout]\""
        n114 = call <vilib>:"Trim Whitespace.vi"("string"=w300) -> ("trimmed string"=w299:string)  [unwired: 1 in]
        n115 = Unbundle By Name(w298) -> ("Verbose?"=w297:bool)
        n116 = case shown="True" w297 {
          tunnel: [w305 w314] -> w302
          tunnel: w301 -> [w305 w313]
          tunnel: w299 -> [_ w312]
          frame False {
          }
          frame True {
            n117 = Empty String/Path?(string/path=w312) -> (empty?=w306:bool)
            n118 = case shown="False" w306 {
              tunnel: w312 -> [w325 _]
              tunnel: [w322 w326] -> w309
              tunnel: [w321 w326] -> w308
              tunnel: [w315 -1] -> w307
              frame False {
                w318 = string[] ["[", "]"] ("delimiters (\\s,\\t,\\r,\\n)")
                n119 = Scan String For Tokens(6:w318, 9:w325) -> (1:w322:string, 2:w324:i32, 3:w323:string)  [unwired: 4 in, 1 out]
                n120 = Scan String For Tokens(6:w318, 8:w324, 9:w323) -> (1:w321:string, 2:w319:i32, 3:w320:string)  [unwired: 3 in, 1 out]
                n121 = Scan String For Tokens(6:w318, 8:w319, 9:w320) -> (1:w317:string)  [unwired: 3 in, 3 out]
                n122 = Decimal String To Number(string=w317, default (0L)=10000 ("Timeout (-1)")) -> (number=w315:i32)  [unwired: 1 in, 1 out]
              }
              frame True {
                w326 = "Important Message" ("token string")
              }
            }
            n123 = call <vilib>:"Init Dialog__lava_lib_ui_tools.vi"("error in (no error)"=w313, "Timeout (-1)"=w307, "Message"=w308, "Dialog Title"=w309) -> ("error out"=w310:errorcluster, "Dialog out"=w311:refnum<class "Dialog__lava_lib_ui_tools.lvclass">)  [unwired: 6 in]
            n124 = while {
              tunnel: w311 -> [w335]
              shift-right: [w333] -> w314
              shift-left: w310 -> [w334]
              stop <- w330 stop-if-true
              n125 = call-dynamic "Dialog Box__lava_lib_ui_tools.vi"("error in (no error)"=w334, "Dialog in"=w335) -> ("error out"=w333:errorcluster, "timed out?"=w329:bool, "Selection"=w332:string)  [unwired: 6 in, 1 out]
              n126 = case shown="\"False\", Default" w332 {
                tunnel: [TRUE FALSE] -> w331
                frame "False", Default {
                }
                frame "True" {
                }
              }
              n127 = Or(x=w331, y=w329) -> (x .or. y?=w330:bool)
              n128 = Wait (ms)(milliseconds to wait=u32 100) -> ()  [unwired: 1 out]
            }
          }
        }
        n129 = call <vilib>:"Add State(s) to Queue__JKI_lib_State_Machine.vi"("State(s) in (\"\")"=w304) -> ("States Out"=w303:string)  [unwired: 14 in]
      }
      frame "---------- Macro ----------" {
        # "Do not put any code in this frame.\n(It is a separator no-op. You can make a copy of this frame to create a new Macro frame)"
        n130 = call <vilib>:"Add State(s) to Queue__JKI_lib_State_Machine.vi"("State(s) in (\"\")"=w341) -> ("States Out"=w340:string)  [unwired: 14 in]
      }
      frame "Macro: Initialize" {
        w342 = string[][] [] ("Hex Table")
        w344 = string[] ["Address", "1", "2", "3", "4"] ("Column Header Strings[]")
        w350 = FALSE ("QUIT")
        w356 = "UI: Initialize\nUI: Front Panel State >> Open\nMacro: Load Config INI\nData: Update"  # UI: Initialize UI: Front Panel State >> Open Macro: Load Config INI Data: Update
        # "Initialization Macro\n(This is called once, when the VI starts)"
        n131 = property on="Hex Table" class="Tbl (strict)"(error in=w348, "Column Headers[]"=w344, "Number of Columns"=u32 5, "Value"=w342) -> (error out=w346:errorcluster)  [unwired: 1 in, 1 out]
        n132 = property on="Bin Table" class="Tbl (strict)"(error in=w346, "Column Headers[]"=w344, "Number of Columns"=u32 5, "Value"=w342) -> (error out=w345:errorcluster)  [unwired: 1 in, 1 out]
        n133 = property on="QUIT" class="Bool (strict)"(error in=w345, "Value"=w350) -> (error out=w352:errorcluster)  [unwired: 1 in, 1 out]
        n134 = property on="Read Device" class="Bool (strict)"(error in=w352, "Value"=w350) -> (error out=w353:errorcluster)  [unwired: 1 in, 1 out]
        n135 = property on="Program Device" class="Bool (strict)"(error in=w353, "Value"=w350) -> (error out=w354:errorcluster)  [unwired: 1 in, 1 out]
        n136 = property on="Write ALL Device" class="Bool (strict)"(error in=w354, "Value"=w350) -> (error out=w355:errorcluster)  [unwired: 1 in, 1 out]
        n137 = property on="Erase ALL Device" class="Bool (strict)"(error in=w355, "Value"=w350) -> (error out=w351:errorcluster)  [unwired: 1 in, 1 out]
        n138 = property on="Help" class="Bool (strict)"(error in=w351, "Value"=w350) -> (error out=w349:errorcluster)  [unwired: 1 in, 1 out]
        n139 = call <vilib>:"Add State(s) to Queue__JKI_lib_State_Machine.vi"("State(s) in Front (\"\")"=w356, "State(s) in (\"\")"=w359) -> ("States Out"=w358:string)  [unwired: 13 in]
      }
      frame "Macro: Exit" {
        # "Exit Macro\n(This is called once, when the VI exits)"
        n140 = Unbundle By Name(w366) -> ("Core.Close Panel on Exit?"=w365:bool)
        n141 = Select(t="UI: Front Panel State >> Close", s=w365, f="") -> (s? t:f=w362:string)
        n142 = call <vilib>:"Add State(s) to Queue__JKI_lib_State_Machine.vi"("State(s) in (\"\")"=w362, "State(s) at Back (\"\")"="Data: Cleanup\nMacro: Save Config INI\nExit") -> ("States Out"=w360:string)  [unwired: 13 in]
        n143 = call <vilib>:"Add State(s) to Queue__JKI_lib_State_Machine.vi"("State(s) in Front (\"\")"=w360, "State(s) in (\"\")"=w369) -> ("States Out"=w368:string)  [unwired: 13 in]
      }
      frame "Macro: Build Hex-Bin Table" {
        w376 = string[][] [] ("array")
        # "Update the Hex strings display post data capture from device"
        n144 = Unbundle By Name(w380) -> ("Read Data"=w379:u8[], "Target Page Size (bytes)"=w370:i32)
        n145 = Array Size(array=w379) -> (size(s)=w378:i32)
        n146 = Quotient & Remainder(x=w378, y=w370) -> (floor(x/y)=w377:i32)  [unwired: 1 out]
        n147 = Increment(x=w377) -> (x+1=w371:i32)
        n148 = for {
          N: w371 -> [_]
          shift-right: [w403] -> _
          shift-left: w379 -> [w402]
          shift-right: [w400] -> w373
          shift-left: w376 -> [w399]
          shift-right: [w391] -> w374
          shift-left: w376 -> [w390]
          tunnel: w370 -> [w386]
          i -> [w384]
          # "Extract n bytes at a time (per page size)\nRemaining elements to shift register"
          n149 = Delete From Array(array=w402, length=w386, index=0) -> (deleted portion=w404:u8[], array with subset deleted=w403:u8[])
          n150 = for {
            tunnel: w404 -> [w419] mode=indexing
            shift-right: [w417] -> _
            shift-left: "" -> [w416]
            shift-right: [w415] -> _
            shift-left: _ -> [w414]
            shift-right: [w411] -> w398
            shift-left: string[] [] ("array") -> [w409]
            shift-right: [w405] -> w393
            shift-left: _ -> [w406]
            i -> [w408]
            w412 = "\t"
            n151 = Number To Hexadecimal String(2:w419) -> (0:w418:string)  [unwired: 1 in]
            n152 = call "Hex_String_to_Binary_String.vi"("bitness"=enum16{"8", "16", "32", "64"}."8", "Hexadecimal String"=w418) -> ("Hex String"=w410:string, "Binary String"=w407:string)  [unwired: 1 in, 1 out]
            n153 = Concatenate Strings(w416, w407, w412) -> (w417:string)
            n154 = Insert Into Array(array=w406, index=w408, new element=w407) -> (w405:string[])
            n155 = Concatenate Strings(w414, w410, w412) -> (w415:string)
            n156 = Insert Into Array(array=w409, index=w408, new element=w410) -> (w411:string[])
          }
          n157 = Number To Hexadecimal String(1:i16 4 ("width (-)"), 2:w384) -> (0:w394:string)
          n158 = Increment(x=w386) -> (x+1=w385:i32)
          n159 = Build Array (concatenate)(w394, w398) -> (w397:string[])
          n160 = Build Array (concatenate)(w394, w393) -> (w395:string[])
          n161 = Reshape Array(w397, w385) -> (w396:string[])
          n162 = Reshape Array(w395, w385) -> (w392:string[])
          n163 = Insert Into Array(array=w390, index (row)=w384, new element=w392) -> (w391:string[][])  [unwired: 1 in]
          n164 = Insert Into Array(array=w399, index (row)=w384, new element=w396) -> (w400:string[][])  [unwired: 1 in]
        }
        n165 = local write "Bin Table"(w374) -> ()
        n166 = local write "Hex Table"(w373) -> ()
        n167 = call <vilib>:"Add State(s) to Queue__JKI_lib_State_Machine.vi"("State(s) in Front (\"\")"="UI: Display Message >>  [Alert!][Hex & Binary Table Parsed][10000]" ("State(s) in Front (\"\")"), "State(s) in (\"\")"=w383) -> ("States Out"=w382:string)  [unwired: 13 in]
        n168 = Bundle By Name(cluster=w380, "Bin Table"=w374, "Hex Table"=w373) -> (w375:T7)
      }
      frame "Macro: Load Binary File" {
        # "Do not put any code in this frame.\n(It is a separator no-op. You can make a copy of this frame to create a new Macro frame)"
        n169 = Unbundle By Name(w424) -> ("Data Address Endianness"=w423:bool)
        n170 = Boolean To (0,1)(Boolean=w423) -> (0, 1=w422:i16)
        n171 = call "File Dialog"("prompt"="Find and Select the Binary or Hex File to Load to EEPROM", "error in"=w429, "pattern (all files)"="*.bin;*.hex") -> ("selected path"=w426:path, "error out"=w425:errorcluster)  [unwired: 9 in, 2 out]
        n172 = Read from Binary File(5:"" ("data type"), 8:w425, 9:w422, 11:w426) -> (0:w420:errorcluster)  [unwired: 2 in, 3 out]
        n173 = call <vilib>:"Add State(s) to Queue__JKI_lib_State_Machine.vi"("State(s) in (\"\")"=w431) -> ("States Out"=w430:string)  [unwired: 14 in]
      }
      frame "Macro: Save Config INI" {
        # "// Save control values & states to INI file\n// Config.INI saved in directory as this VI"
        n174 = Unbundle By Name(w437) -> ("INI Path"=w436:path)
        n175 = control-ref of="This VI"() -> (w438:refnum<vi>)
        n176 = call "Utility Write Config INI to File.vi"("File Type"=".ini", "Error In"=w441, "reference"=w438, "Path In"=w436) -> ("Error Out"=w440:errorcluster, "Path Out"=w435:path)  [unwired: 6 in]
        n177 = Path To String(path=w435) -> (string=w433:string)
        n178 = Format Into String(format string="UI: Display Message >> [Configuration INI Saved To PATH: ][%s][10000]" ("State(s) in Front (\"\")"), w433) -> (resulting string=w432:string)  [unwired: 2 in, 1 out]
        n179 = call <vilib>:"Add State(s) to Queue__JKI_lib_State_Machine.vi"("State(s) in Front (\"\")"=w432, "State(s) in (\"\")"=w443) -> ("States Out"=w442:string)  [unwired: 13 in]
      }
      frame "Macro: Load Config INI" {
        n180 = Unbundle By Name(w446) -> ("INI Path"=w445:path)
        n181 = control-ref of="This VI"() -> (w453:refnum<vi>)
        n182 = call "Utility Load Config INI from File.vi"("File Type"=".ini", "Error In"=w450, "reference"=w453, "Path In"=w445) -> ("Error Out"=w449:errorcluster, "Path Out"=w452:path)  [unwired: 6 in]
        n183 = Path To String(path=w452) -> (string=w447:string)
        n184 = Format Into String(format string="UI: Display Message >> [Configuration INI Loaded From PATH: ][%s][10000]" ("State(s) in Front (\"\")"), w447) -> (resulting string=w444:string)  [unwired: 2 in, 1 out]
        n185 = call <vilib>:"Add State(s) to Queue__JKI_lib_State_Machine.vi"("State(s) in Front (\"\")"=w444, "State(s) in (\"\")"=w455) -> ("States Out"=w454:string)  [unwired: 13 in]
      }
      frame "---------- NI8451: Template ----------" {
        # "Template Separator\n(You can make a copy of, or modify, this frame)"
        n186 = call <vilib>:"Add State(s) to Queue__JKI_lib_State_Machine.vi"("State(s) in (\"\")"=w459) -> ("States Out"=w458:string)  [unwired: 14 in]
      }
      frame "93LC56BT Notes" {
        # "Template Separator\n(You can make a copy of, or modify, this frame)"
        n187 = call <vilib>:"Add State(s) to Queue__JKI_lib_State_Machine.vi"("State(s) in (\"\")"=w463) -> ("States Out"=w462:string)  [unwired: 14 in]
      }
      frame "93C86 Notes" {
        # "Microchip 93C76/86 8K/16K 5.0V Microwire Serial EEPROM"
        n188 = disable-structure shown="Enabled" {
          frame Enabled {
          }
          frame Disabled {
          }
          frame Disabled {
          }
        }
      }
      frame "NI8451: Prep EEPROM Data" {
        (unwired) u16[][] [[65281, 21], [8193, 417], [65281, 0], [4609, 43690]]
        # "Template Separator\n(You can make a copy of, or modify, this frame)"
        n189 = call <vilib>:"Add State(s) to Queue__JKI_lib_State_Machine.vi"("State(s) in (\"\")"=w470) -> ("States Out"=w469:string)  [unwired: 14 in]
      }
      frame "NI8451: Device Mode" {
        # "Send Message if Mode is not yet supported\nCommand Format:  \"UI: Display Message >> [Window Title] [Message] [Timeout]\""
        n190 = Unbundle By Name(w474) -> ("Device Mode"=w473:enum16{"SPI", "I2C", "DIO"})
        n191 = case shown="\"DIO\"" w473 {
          tunnel: [w477 "UI: Display Message >>  [Alert!][I2C Mode is NOT supported at this time][10000]\n" "UI: Display Message >>  [Alert!][DIO Mode is NOT supported at this time][10000]\n"] -> w471
          tunnel: w472 -> [w477 _ _]
          frame "SPI", Default {
          }
          frame "I2C" {
          }
          frame "DIO" {
          }
        }
        n192 = call <vilib>:"Add State(s) to Queue__JKI_lib_State_Machine.vi"("State(s) in (\"\")"=w471) -> ("States Out"=w476:string)  [unwired: 14 in]
      }
      frame "NI8451: Init SPI" {
        # "The Microchip EEPROMs' CS idle\nstate is LOW and asserted HIGH\nso set SPI to LOW post INIT."
        # "Step 1: Set the I/O reference voltage:\n\nNot all NI-845x hardware support all voltage levels. \nPlease consult your hardware documentation for more information.\n\nStep 2: Create the script and configure the SPI bus:\n\na) Create the script\nb) Switch the SPI bus pins into master mode. \n    This automatically sets all CS lines to be high.\nc) Configure the Phase and Plarity to mode 0, in \n    which the polarity and phase are both set to \n    zero, however this may be configured for \n    other EEPROMs. \nd) Configure the Clock rate as set by the front \n    panel control."
        n193 = Unbundle By Name(w491) -> ("CS/SS"=w486:u32, "CLK Rate (kHz)"=w487:u16, "NI8451 Device ID"=w490:T2, "IO Level (V)"=w489:i32, "CLK Polarity (CPOL)"=w483:i32, "CLK Phase (CPHS)"=w482:i32, "CS Idle Level"=w484:enum16{"Low (Assert High)", "High (Assert Low)"})
        n194 = property on="Property Node" class="NI-845x Device"(reference=w490, error in=w485, "IoVoltLevel"=w489) -> (error out=w495:errorcluster)  [unwired: 1 out]
        n195 = call <vilib>:"NI-845x SPI Create Script Reference.vi"("error in (no error)"=w495) -> ("error out"=w494:errorcluster, "spi script reference"=w488:T4)  [unwired: 9 out]
        n196 = call <vilib>:"NI-845x SPI Script Enable SPI.vi"("error in (no error)"=w494, "spi script reference in"=w488) -> ("error out"=w496:errorcluster, "spi script reference out"=w497:T4)  [unwired: 8 out]
        n197 = Bundle By Name(cluster=w491, "SPI Script Reference"=w488) -> (w480:T7)
        n198 = call <vilib>:"NI-845x SPI Script Clock Polarity Phase.vi"("error in (no error)"=w496, "clock phase (0)"=w482, "clock polarity (0)"=w483, "spi script reference in"=w497) -> ("error out"=w492:errorcluster, "spi script reference out"=w493:T4)  [unwired: 2 in, 4 out]
        n199 = call <vilib>:"NI-845x SPI Script Clock Rate.vi"("error in (no error)"=w492, "clock rate in kHz (1000)"=w487, "spi script reference in"=w493) -> ("error out"=w498:errorcluster, "spi script reference out"=w499:T4)  [unwired: 1 in, 6 out]
        n200 = case shown="\"Low (Assert High)\"" w484 {
          tunnel: w499 -> [w506 w511]
          tunnel: w498 -> [w505 w510]
          tunnel: w486 -> [w504 w509]
          tunnel: [w503 w508] -> w481
          tunnel: [w502 w507] -> _
          frame "Low (Assert High)" {
            n201 = call <vilib>:"NI-845x SPI Script CS Low.vi"("error in (no error)"=w505, "chip select (0)"=w504, "spi script reference in"=w506) -> ("error out"=w503:errorcluster, "spi script reference out"=w502:T4)  [unwired: 7 in]
          }
          frame "High (Assert Low)" {
            n202 = call <vilib>:"NI-845x SPI Script CS High.vi"("error in (no error)"=w510, "chip select (0)"=w509, "spi script reference in"=w511) -> ("error out"=w508:errorcluster, "spi script reference out"=w507:T4)  [unwired: 7 in]
          }
        }
        n203 = call <vilib>:"Add State(s) to Queue__JKI_lib_State_Machine.vi"("State(s) in (\"\")"=w501) -> ("States Out"=w500:string)  [unwired: 14 in]
      }
      frame "NI8451: EWEN" {
        # "The Microchip 93C86 CS idle\nstate is LOW and asserted HIGH"
        # "1. Send SB & EWEN Opcode for 93LC56BT\n2. A dummy address byte\n3. A dummy data byte"
        n204 = Unbundle By Name(w517) -> ("EEPROM Device Type"=w512:enum16{"Microchip 93C86", "Microchip LC56BT"}, "EWEN"=w514:u8, "SPI Script Reference"=w516:T4, "CS/SS"=w513:u32, "CS Idle Level"=w515:enum16{"Low (Assert High)", "High (Assert Low)"})
        n205 = case shown="\"Microchip 93C86\"" w512 {
          tunnel: [w528 w533] -> w524
          tunnel: w514 -> [w527 w532]
          frame "Microchip LC56BT" {
            w529 = u8 0
            # "16-bit Data & 8-bit Address"
            n206 = Build Array(w527, w529, w529) -> (w528:u8[])
          }
          frame "Microchip 93C86" {
            w531 = u16 0
            # "16-bit Data & Address"
            n207 = To Unsigned Word Integer(number=w532) -> (unsigned 16bit integer=w530:u16)
            n208 = Build Array(w530, w531, w531) -> (w533:u16[])
          }
        }
        n209 = case shown="\"Low (Assert High)\"" w515 {
          tunnel: [w546 w551] -> w521
          tunnel: [w545 w550] -> w520
          tunnel: w519 -> [w544 w549]
          tunnel: w516 -> [w543 w548]
          tunnel: w513 -> [w542 w547]
          frame "Low (Assert High)" {
            n210 = call <vilib>:"NI-845x SPI Script CS High.vi"("error in (no error)"=w544, "chip select (0)"=w542, "spi script reference in"=w543) -> ("error out"=w545:errorcluster, "spi script reference out"=w546:T4)  [unwired: 7 in]
          }
          frame "High (Assert Low)", Default {
            n211 = call <vilib>:"NI-845x SPI Script CS Low.vi"("error in (no error)"=w549, "chip select (0)"=w547, "spi script reference in"=w548) -> ("error out"=w550:errorcluster, "spi script reference out"=w551:T4)  [unwired: 7 in]
          }
        }
        n212 = call <vilib>:"NI-845x SPI Script Write Read.vi"("error in (no error)"=w520, "write data"=w524, "spi script reference in"=w521) -> ("error out"=w522:errorcluster, "spi script reference out"=w523:T4)  [unwired: 1 in, 6 out]
        n213 = case shown="\"Low (Assert High)\"" w515 {
          tunnel: w523 -> [w537 w541]
          tunnel: w522 -> [w536 w540]
          tunnel: [w535 w539] -> w518
          tunnel: w513 -> [w534 w538]
          frame "High (Assert Low)" {
            n214 = call <vilib>:"NI-845x SPI Script CS High.vi"("error in (no error)"=w536, "chip select (0)"=w534, "spi script reference in"=w537) -> ("error out"=w535:errorcluster)  [unwired: 7 in, 1 out]
          }
          frame "Low (Assert High)" {
            n215 = call <vilib>:"NI-845x SPI Script CS Low.vi"("error in (no error)"=w540, "chip select (0)"=w538, "spi script reference in"=w541) -> ("error out"=w539:errorcluster)  [unwired: 7 in, 1 out]
          }
        }
        n216 = call <vilib>:"Add State(s) to Queue__JKI_lib_State_Machine.vi"("State(s) in (\"\")"=w526) -> ("States Out"=w525:string)  [unwired: 14 in]
      }
      frame "NI8451: READ 93LC56BT" {
        # "For Microchip LC56BT the MSB is transmitted first (high endian)\nThe Microchip LC56BT CS idle state is LOW and asserted HIGH"
        n217 = Unbundle By Name(w569) -> ("CS/SS"=w570:u32, "CS Idle Level"=w566:enum16{"Low (Assert High)", "High (Assert Low)"}, "SPI Script Reference"=w571:T4, "READ"=w567:u8, "EEPROM Address (u8)"=w562:u16, "Number of Bytes (Read)"=w556:i16)
        n218 = case shown="\"Low (Assert High)\"" w566 {
          tunnel: [w592 w597] -> w573
          tunnel: [w591 w596] -> w572
          tunnel: w571 -> [w590 w595]
          tunnel: w570 -> [w589 w594]
          tunnel: w568 -> [w588 w593]
          frame "High (Assert Low)", Default {
            n219 = call <vilib>:"NI-845x SPI Script CS Low.vi"("error in (no error)"=w588, "chip select (0)"=w589, "spi script reference in"=w590) -> ("error out"=w592:errorcluster, "spi script reference out"=w591:T4)  [unwired: 7 in]
          }
          frame "Low (Assert High)" {
            n220 = call <vilib>:"NI-845x SPI Script CS High.vi"("error in (no error)"=w593, "chip select (0)"=w594, "spi script reference in"=w595) -> ("error out"=w597:errorcluster, "spi script reference out"=w596:T4)  [unwired: 7 in]
          }
        }
        n221 = Initialize Array(u16 255 ("element"), w556) -> (w553:u16[])
        n222 = To Unsigned Byte Integer(number=w567) -> (unsigned 8bit integer=w555:u8)
        n223 = To Unsigned Byte Integer(number=w562) -> (unsigned 8bit integer=w554:u8)
        n224 = Build Array (concatenate)(w555, w554, w553) -> (w563:u16[])
        n225 = call <vilib>:"NI-845x SPI Script Write Read.vi"("error in (no error)"=w573, "write data"=w563, "spi script reference in"=w572) -> ("error out"=w575:errorcluster, "script read index"=w564:u32, "spi script reference out"=w574:T4)  [unwired: 1 in, 5 out]
        n226 = Bundle By Name(cluster=w569, "script read index"=w564) -> (w565:T7)
        n227 = case shown="\"High (Assert Low)\", Default" w566 {
          tunnel: w575 -> [w582 w587]
          tunnel: w574 -> [w581 w586]
          tunnel: w570 -> [w580 w585]
          tunnel: [w579 w584] -> w559
          tunnel: [w578 w583] -> w558
          frame "High (Assert Low)", Default {
            n228 = call <vilib>:"NI-845x SPI Script CS High.vi"("error in (no error)"=w582, "chip select (0)"=w580, "spi script reference in"=w581) -> ("error out"=w579:errorcluster, "spi script reference out"=w578:T4)  [unwired: 7 in]
          }
          frame "Low (Assert High)" {
            n229 = call <vilib>:"NI-845x SPI Script CS Low.vi"("error in (no error)"=w587, "chip select (0)"=w585, "spi script reference in"=w586) -> ("error out"=w584:errorcluster, "spi script reference out"=w583:T4)  [unwired: 7 in]
          }
        }
        n230 = Multiply(x=u32 1 ("delay in microseconds (0)"), y=w556) -> (x*y=w561:u32)
        n231 = call-poly <vilib>:"NI-845x SPI Script Delay.vi"("error in (no error)"=w559, "delay in microseconds (0)"=w561, "spi script reference in"=w558) -> ("error out"=w557:errorcluster)  [unwired: 7 in, 1 out]
        n232 = call <vilib>:"Add State(s) to Queue__JKI_lib_State_Machine.vi"("State(s) in (\"\")"=w577) -> ("States Out"=w576:string)  [unwired: 14 in]
      }
      frame "NI8451: WRITE 93LC56BT" {
        # "For 93LC56BT the MSB is transmitted first (high endian)\nThe Microchip 93LC56BT CS idle state is LOW and asserted HIGH\nThe Microchip 93LC56BT  has 128x16-bit organization (ORG not connected)"
        n233 = Unbundle By Name(w607) -> ("CS/SS"=w602:u32, "Page Write Delay (ms)"=w600:u8, "SPI Script Reference"=w606:T4, "WRITE"=w603:u8, "EEPROM Program Data"=w598:string[][])  [unwired: 1 out]
        n234 = disable-structure shown="Disabled" {
          frame Disabled {
            (unwired) u8 170 ("element")
            (unwired) u8 187 ("element")
            (unwired) u8 2 ("element")
            n235 = Number To Boolean Array() -> ()  [unwired: 1 in, 1 out]
            n236 = Reverse 1D Array() -> ()  [unwired: 1 in, 1 out]
            n237 = Boolean Array To Number() -> ()  [unwired: 1 in, 1 out]
          }
          frame Enabled {
          }
        }
        n238 = for {
          tunnel: w608 -> [w629]
          tunnel: w606 -> [w628]
          tunnel: [w653] -> w604
          tunnel: w603 -> [w652]
          tunnel: w602 -> [w631]
          tunnel: [w630] -> w601
          tunnel: w600 -> [w625]
          tunnel: w598 -> [w618] mode=indexing
          # "Note: the NI-8451 can only send 8 bits at a time"
          # "Data"
          # "Address"
          # "Tcsl"
          n239 = call-poly <vilib>:"NI-845x SPI Script Delay.vi"("error in (no error)"=w629, "delay in milliseconds (0)"=w625, "spi script reference in"=w628) -> ("error out"=w626:errorcluster, "spi script reference out"=w627:T4)  [unwired: 7 out]
          n240 = Index Array(array=w618, index=0) -> (element=w621:string)
          n241 = Index Array(array=w618, index=1) -> (element=w624:string)
          n242 = call "Hex_String_to_Binary_String.vi"("bitness"=enum16{"8", "16", "32", "64"}."8", "Hexadecimal String"=w621) -> ("number"=w617:u64)  [unwired: 1 in, 2 out]
          n243 = call "Hex_String_to_Binary_String.vi"("bitness"=enum16{"8", "16", "32", "64"}."16", "Hexadecimal String"=w624) -> ("number"=w616:u64)  [unwired: 1 in, 2 out]
          n244 = To Unsigned Byte Integer(number=w617) -> (unsigned 8bit integer=w612:u8)
          n245 = To Unsigned Word Integer(number=w616) -> (unsigned 16bit integer=w615:u16)
          n246 = Split Number(x=w615) -> (hi(x)=w614:u8, lo(x)=w613:u8)
          n247 = To Unsigned Byte Integer(number=w652) -> (unsigned 8bit integer=w611:u8)
          n248 = call <vilib>:"NI-845x SPI Script CS High.vi"("error in (no error)"=w626, "chip select (0)"=w631, "spi script reference in"=w627) -> ("error out"=w643:errorcluster, "spi script reference out"=w644:T4)  [unwired: 7 in]
          n249 = Build Array(w611, w612, w614, w613) -> (w642:u8[])
          n250 = call <vilib>:"NI-845x SPI Script Write Read.vi"("error in (no error)"=w643, "write data"=w642, "spi script reference in"=w644) -> ("error out"=w651:errorcluster, "script read index"=w653:u32, "spi script reference out"=w650:T4)  [unwired: 1 in, 5 out]
          n251 = Array Subset(array=w642, index=2) -> (w640:u8[])  [unwired: 1 in]
          n252 = call <vilib>:"NI-845x SPI Script CS Low.vi"("error in (no error)"=w651, "chip select (0)"=w631, "spi script reference in"=w650) -> ("error out"=w649:errorcluster, "spi script reference out"=w648:T4)  [unwired: 7 in]
          n253 = local write "Data Bytes Written"(w640) -> ()
          n254 = call-poly <vilib>:"NI-845x SPI Script Delay.vi"("error in (no error)"=w649, "delay in microseconds (0)"=u16 1, "spi script reference in"=w648) -> ("error out"=w646:errorcluster, "spi script reference out"=w645:T4)  [unwired: 7 out]
          n255 = call <vilib>:"NI-845x SPI Script CS High.vi"("error in (no error)"=w646, "chip select (0)"=w631, "spi script reference in"=w645) -> ("error out"=w637:errorcluster, "spi script reference out"=w639:T4)  [unwired: 7 in]
          n256 = call-poly <vilib>:"NI-845x SPI Script Delay.vi"("error in (no error)"=w637, "delay in microseconds (0)"=u16 100, "spi script reference in"=w639) -> ("spi script reference out"=w636:T4)  [unwired: 8 out]
          n257 = call <vilib>:"NI-845x SPI Script CS Low.vi"("error in (no error)"=w637, "chip select (0)"=w631, "spi script reference in"=w636) -> ("error out"=w635:errorcluster, "spi script reference out"=w634:T4)  [unwired: 7 in]
          n258 = call <vilib>:"NI-845x SPI Script CS High.vi"("error in (no error)"=w635, "chip select (0)"=w631, "spi script reference in"=w634) -> ("error out"=w633:errorcluster, "spi script reference out"=w632:T4)  [unwired: 7 in]
          n259 = call <vilib>:"NI-845x SPI Script CS Low.vi"("error in (no error)"=w633, "chip select (0)"=w631, "spi script reference in"=w632) -> ("error out"=w630:errorcluster)  [unwired: 7 in, 1 out]
        }
        n260 = Bundle By Name(cluster=w607, "script read index"=w604) -> (w605:T7)
        n261 = call <vilib>:"Add State(s) to Queue__JKI_lib_State_Machine.vi"("State(s) in (\"\")"=w610, "State(s) at Back (\"\")"="UI: Display Message >>  [Alert!][WRITE Data Completed][10000]" ("State(s) in Front (\"\")")) -> ("States Out"=w609:string)  [unwired: 13 in]
      }
      frame "NI8451: READ 93C86" {
        # "~0.25ns per word"
        # "For Microchip 93C86 the MSB is transmitted first (high endian)\nThe Microchip 93C86 CS idle state is LOW and asserted HIGH\nThis node needs the NI8452 model. NI8451 only supports 8 bits"
        n262 = Unbundle By Name(w671) -> ("CS/SS"=w672:u32, "CS Idle Level"=w669:enum16{"Low (Assert High)", "High (Assert Low)"}, "SPI Script Reference"=w656:T4, "READ"=w670:u8, "EEPROM Address (u8)"=w665:u16, "Number of Bytes (Read)"=w654:i16)
        n263 = To Unsigned Word Integer(number=w665) -> (unsigned 16bit integer=w663:u16)
        n264 = case shown="\"8 bits\"" enum16{"8 bits", "16 bits"}."8 bits" ("Address Width") {
          tunnel: w663 -> [w683 w700]
          tunnel: [w694 w698] -> w666
          tunnel: w670 -> [w693 w699]
          tunnel: w665 -> [w684 _]
          tunnel: w654 -> [w679 w696]
          frame "8 bits" {
            n265 = Number To Boolean Array(number=w684) -> (Boolean array=w686:bool[])
            n266 = Number To Boolean Array(number=w693) -> (Boolean array=w692:bool[])
            n267 = Split Number(x=w683) -> (hi(x)=w682:u8, lo(x)=w681:u8)
            n268 = Index Array(array=w686, index=8) -> (element=w685:bool)
            n269 = Initialize Array(u8 255 ("element"), w679) -> (w678:u8[])
            n270 = Replace Array Subset(array=w692, new element=w685, index=3) -> (w690:bool[])
            n271 = Boolean Array To Number(Boolean array=w690) -> (number=w689:u32)
            n272 = To Unsigned Byte Integer(number=w689) -> (unsigned 8bit integer=w688:u8)
            n273 = Build Array (concatenate)(w688, w682, w681, w678) -> (w694:u8[])
          }
          frame "16 bits", Default {
            n274 = Split Number(x=w700) -> (hi(x)=w702:u8, lo(x)=w701:u8)
            n275 = Initialize Array(u16 255 ("element"), w696) -> (w695:u16[])
            n276 = Build Array (concatenate)(w699, w702, w701, w695) -> (w698:u16[])
          }
        }
        n277 = case shown="\"Low (Assert High)\"" w669 {
          tunnel: [w717 w722] -> w655
          tunnel: [w716 w721] -> w673
          tunnel: w656 -> [w715 w720]
          tunnel: w672 -> [w714 w719]
          tunnel: w657 -> [w713 w718]
          frame "High (Assert Low)", Default {
            n278 = call <vilib>:"NI-845x SPI Script CS Low.vi"("error in (no error)"=w713, "chip select (0)"=w714, "spi script reference in"=w715) -> ("error out"=w717:errorcluster, "spi script reference out"=w716:T4)  [unwired: 7 in]
          }
          frame "Low (Assert High)" {
            n279 = call <vilib>:"NI-845x SPI Script CS High.vi"("error in (no error)"=w718, "chip select (0)"=w719, "spi script reference in"=w720) -> ("error out"=w722:errorcluster, "spi script reference out"=w721:T4)  [unwired: 7 in]
          }
        }
        n280 = call <vilib>:"NI-845x SPI Script Write Read.vi"("error in (no error)"=w655, "write data"=w666, "spi script reference in"=w673) -> ("error out"=w675:errorcluster, "script read index"=w667:u32, "spi script reference out"=w674:T4)  [unwired: 1 in, 5 out]
        n281 = case shown="\"Low (Assert High)\"" w669 {
          tunnel: w675 -> [w707 w712]
          tunnel: w674 -> [w706 w711]
          tunnel: w672 -> [w705 w710]
          tunnel: [w704 w709] -> w662
          tunnel: [w703 w708] -> w660
          frame "High (Assert Low)", Default {
            n282 = call <vilib>:"NI-845x SPI Script CS High.vi"("error in (no error)"=w707, "chip select (0)"=w705, "spi script reference in"=w706) -> ("error out"=w704:errorcluster, "spi script reference out"=w703:T4)  [unwired: 7 in]
          }
          frame "Low (Assert High)" {
            n283 = call <vilib>:"NI-845x SPI Script CS Low.vi"("error in (no error)"=w712, "chip select (0)"=w710, "spi script reference in"=w711) -> ("error out"=w709:errorcluster, "spi script reference out"=w708:T4)  [unwired: 7 in]
          }
        }
        n284 = Bundle By Name(cluster=w671, "script read index"=w667) -> (w668:T7)
        n285 = Quotient & Remainder(x=w654, y=u32 4 ("delay in microseconds (0)")) -> (floor(x/y)=w659:u32)  [unwired: 1 out]
        n286 = call-poly <vilib>:"NI-845x SPI Script Delay.vi"("error in (no error)"=w662, "delay in microseconds (0)"=w659, "spi script reference in"=w660) -> ("error out"=w661:errorcluster)  [unwired: 7 in, 1 out]
        n287 = call <vilib>:"Add State(s) to Queue__JKI_lib_State_Machine.vi"("State(s) in (\"\")"=w677) -> ("States Out"=w676:string)  [unwired: 14 in]
      }
      frame "NI8451: WRITE 93C86" {
        # "Index EEPROM\nProgram Data\nper row"
        # "For MC93C86 the MSB is transmitted first (high endian)\nThe Microchip 93C86 CS idle state is LOW and asserted HIGH\nThis node needs the NI8452 model. NI8451 only supports 8 bits"
        n288 = Unbundle By Name(w732) -> ("CS/SS"=w727:u32, "Page Write Delay (ms)"=w725:u8, "SPI Script Reference"=w731:T4, "WRITE"=w728:u8, "EEPROM Program Data"=w724:string[][])
        n289 = for {
          tunnel: w733 -> [w770]
          tunnel: w731 -> [w769]
          tunnel: [w768] -> w729
          tunnel: w728 -> [w767]
          tunnel: w727 -> [w766]
          tunnel: [w765] -> w726
          tunnel: w725 -> [w764]
          tunnel: w724 -> [w744] mode=indexing
          # "Data"
          # "Address"
          n290 = Index Array(array=w744, index=0) -> (element=w746:string)
          n291 = Index Array(array=w744, index=1) -> (element=w742:string)
          n292 = call-poly <vilib>:"NI-845x SPI Script Delay.vi"("error in (no error)"=w770, "delay in milliseconds (0)"=w764, "spi script reference in"=w769) -> ("error out"=w736:errorcluster, "spi script reference out"=w737:T4)  [unwired: 7 out]
          n293 = call "Hex_String_to_Binary_String.vi"("bitness"=enum16{"8", "16", "32", "64"}."16", "Hexadecimal String"=w746) -> ("number"=w740:u64)  [unwired: 1 in, 2 out]
          n294 = call "Hex_String_to_Binary_String.vi"("bitness"=enum16{"8", "16", "32", "64"}."16", "Hexadecimal String"=w742) -> ("number"=w741:u64)  [unwired: 1 in, 2 out]
          n295 = Split Number(x=w741) -> (hi(x)=w755:u32, lo(x)=w754:u32)
          n296 = case shown="\"16 bits\", Default" enum16{"8 bits", "16 bits"}."16 bits" ("Address Width") {
            tunnel: [w783 w787] -> w759
            tunnel: w740 -> [w771 _]
            tunnel: w767 -> [w777 w788]
            tunnel: w755 -> [w773 _]
            tunnel: w754 -> [w772 _]
            tunnel: w741 -> [_ w784]
            tunnel: w740 -> [_ w786]
            frame "8 bits" {
              n297 = Number To Boolean Array(number=w777) -> (Boolean array=w782:bool[])
              n298 = Number To Boolean Array(number=w771) -> (Boolean array=w776:bool[])
              n299 = Index Array(array=w776, index=8) -> (element=w774:bool)
              n300 = Replace Array Subset(array=w782, new element=w774, index=3) -> (w780:bool[])
              n301 = Boolean Array To Number(Boolean array=w780) -> (number=w779:u32)
              n302 = To Unsigned Byte Integer(number=w779) -> (unsigned 8bit integer=w778:u8)
              n303 = Build Array(w778, w771, w773, w772) -> (w783:u64[])
            }
            frame "16 bits", Default {
              n304 = To Unsigned Word Integer(number=w788) -> (unsigned 16bit integer=w785:u16)
              n305 = Build Array(w785, w786, w784, w784) -> (w787:u64[])
            }
          }
          n306 = call <vilib>:"NI-845x SPI Script CS High.vi"("error in (no error)"=w736, "chip select (0)"=w766, "spi script reference in"=w737) -> ("error out"=w760:errorcluster, "spi script reference out"=w761:T4)  [unwired: 7 in]
          n307 = call <vilib>:"NI-845x SPI Script Write Read.vi"("error in (no error)"=w760, "write data"=w759, "spi script reference in"=w761) -> ("error out"=w763:errorcluster, "script read index"=w768:u32, "spi script reference out"=w762:T4)  [unwired: 1 in, 5 out]
          n308 = Array Subset(array=w759, index=0) -> (w757:u64[])  [unwired: 1 in]
          n309 = local write "Data Bytes Written"(w757) -> ()
          n310 = call <vilib>:"NI-845x SPI Script CS Low.vi"("error in (no error)"=w763, "chip select (0)"=w766, "spi script reference in"=w762) -> ("error out"=w738:errorcluster, "spi script reference out"=w739:T4)  [unwired: 7 in]
          n311 = call <vilib>:"NI-845x SPI Script CS High.vi"("error in (no error)"=w738, "chip select (0)"=w766, "spi script reference in"=w739) -> ("error out"=w753:errorcluster, "spi script reference out"=w751:T4)  [unwired: 7 in]
          n312 = call-poly <vilib>:"NI-845x SPI Script Delay.vi"("error in (no error)"=w753, "delay in microseconds (0)"=u16 2, "spi script reference in"=w751) -> ("error out"=w752:errorcluster, "spi script reference out"=w750:T4)  [unwired: 7 out]
          n313 = call <vilib>:"NI-845x SPI Script CS Low.vi"("error in (no error)"=w752, "chip select (0)"=w766, "spi script reference in"=w750) -> ("error out"=w765:errorcluster)  [unwired: 7 in, 1 out]
        }
        n314 = Bundle By Name(cluster=w732, "script read index"=w729) -> (w730:T7)
        n315 = call <vilib>:"Add State(s) to Queue__JKI_lib_State_Machine.vi"("State(s) in (\"\")"=w735, "State(s) at Back (\"\")"="UI: Display Message >>  [Alert!][WRITE Data Completed][10000]" ("State(s) in Front (\"\")")) -> ("States Out"=w734:string)  [unwired: 13 in]
      }
      frame "NI8451: READ [RESERVED]" {
        # "This is reserved for a generic EEPROM with data paging capability\n** Use this as a template for other EEPROM device types **\nSEE DEVICE DATA SHEET FOR TIMING INFORMATION"
        n316 = Unbundle By Name(w801) -> ("CS/SS"=w802:u32, "CS Idle Level"=w796:enum16{"Low (Assert High)", "High (Assert Low)"}, "SPI Script Reference"=w803:T4, "Address Width"=w793:enum16{"8 bits", "16 bits"}, "READ"=w797:u8, "Data Address Endianness"=w798:bool, "EEPROM Address (u8)"=w791:u16, "Number of Bytes (Read)"=w792:i16, "Target Page Size (bytes)"=w790:i32)
        n317 = call "CreateWriteCluster.vi"("Page Size in Bytes"=w790, "EEPROM Starting Address"=w791, "Number of Bytes to Write"=w792) -> ("Array of Write Cluster Information"=w789:T9)  [unwired: 1 in]
        n318 = for {
          tunnel: w803 -> [w824]
          tunnel: w802 -> [w823]
          tunnel: w800 -> [w822]
          tunnel: [w821] -> w799
          tunnel: w798 -> [w820]
          tunnel: w797 -> [w819]
          tunnel: w796 -> [w818]
          tunnel: [w817] -> w794
          tunnel: w793 -> [w810]
          tunnel: w789 -> [w809] mode=indexing
          n319 = case shown="\"Low (Assert High)\"" w818 {
            tunnel: [w864 w869] -> w826
            tunnel: [w863 w868] -> w825
            tunnel: w824 -> [w862 w867]
            tunnel: w823 -> [w861 w866]
            tunnel: w822 -> [w860 w865]
            frame "High (Assert Low)", Default {
              n320 = call <vilib>:"NI-845x SPI Script CS Low.vi"("error in (no error)"=w860, "chip select (0)"=w861, "spi script reference in"=w862) -> ("error out"=w864:errorcluster, "spi script reference out"=w863:T4)  [unwired: 7 in]
            }
            frame "Low (Assert High)" {
              n321 = call <vilib>:"NI-845x SPI Script CS High.vi"("error in (no error)"=w865, "chip select (0)"=w866, "spi script reference in"=w867) -> ("error out"=w869:errorcluster, "spi script reference out"=w868:T4)  [unwired: 7 in]
            }
          }
          n322 = Unbundle By Name(w809) -> ("EEPROM Address"=w806:u16, "Data Index"=w807:u32, "Length"=w808:u32)
          n323 = Select(t=i16 0, s=w820, f=i16 -8) -> (s? t:f=w813:i16)
          n324 = Rotate(1:w806, 2:w813) -> (0:w812:u16)
          n325 = Initialize Array(w807, w808) -> (w811:u32[])
          n326 = case shown="\"8 bits\"" w810 {
            tunnel: w812 -> [w844 w849]
            tunnel: [w845 w847] -> w816
            tunnel: w819 -> [w839 w848]
            tunnel: w820 -> [w840 _]
            tunnel: w811 -> [w829 w846]
            tunnel: w806 -> [w830 _]
            frame "8 bits" {
              n327 = Number To Boolean Array(number=w830) -> (Boolean array=w832:bool[])
              n328 = Number To Boolean Array(number=w839) -> (Boolean array=w838:bool[])
              n329 = Split Number(x=w844) -> (hi(x)=w842:u8, lo(x)=w843:u8)
              n330 = Index Array(array=w832, index=8) -> (element=w831:bool)
              n331 = Replace Array Subset(array=w838, new element=w831, index=3) -> (w836:bool[])
              n332 = Select(t=w843, s=w840, f=w842) -> (s? t:f=w841:u8)
              n333 = Boolean Array To Number(Boolean array=w836) -> (number=w835:u32)
              n334 = To Unsigned Byte Integer(number=w835) -> (unsigned 8bit integer=w834:u8)
              n335 = Build Array (concatenate)(w834, w841, w829) -> (w845:u32[])
            }
            frame "16 bits", Default {
              n336 = Split Number(x=w849) -> (hi(x)=w851:u8, lo(x)=w850:u8)
              n337 = Build Array (concatenate)(w848, w851, w850, w846) -> (w847:u32[])
            }
          }
          n338 = call <vilib>:"NI-845x SPI Script Write Read.vi"("error in (no error)"=w826, "write data"=w816, "spi script reference in"=w825) -> ("error out"=w828:errorcluster, "script read index"=w817:u32, "spi script reference out"=w827:T4)  [unwired: 1 in, 5 out]
          n339 = case shown="\"Low (Assert High)\"" w818 {
            tunnel: w828 -> [w855 w859]
            tunnel: w827 -> [w854 w858]
            tunnel: w823 -> [w853 w857]
            tunnel: [w852 w856] -> w821
            frame "High (Assert Low)", Default {
              n340 = call <vilib>:"NI-845x SPI Script CS High.vi"("error in (no error)"=w855, "chip select (0)"=w853, "spi script reference in"=w854) -> ("error out"=w852:errorcluster)  [unwired: 7 in, 1 out]
            }
            frame "Low (Assert High)" {
              n341 = call <vilib>:"NI-845x SPI Script CS Low.vi"("error in (no error)"=w859, "chip select (0)"=w857, "spi script reference in"=w858) -> ("error out"=w856:errorcluster)  [unwired: 7 in, 1 out]
            }
          }
        }
        n342 = Bundle By Name(cluster=w801, "script read index"=w794) -> (w795:T7)
        n343 = call <vilib>:"Add State(s) to Queue__JKI_lib_State_Machine.vi"("State(s) in (\"\")"=w805) -> ("States Out"=w804:string)  [unwired: 14 in]
      }
      frame "NI8451: WRITE  [RESERVED]" {
        # "This is reserved for a generic EEPROM with data paging capability\n** Use this as a template for other EEPROM device types **\nSEE DEVICE DATA SHEET FOR TIMING INFORMATION"
        n344 = Unbundle By Name(w886) -> ("CS/SS"=w877:u32, "CS Idle Level"=w878:enum16{"Low (Assert High)", "High (Assert Low)"}, "Address Width"=w876:enum16{"8 bits", "16 bits"}, "Page Write Delay (ms)"=w884:u8, "SPI Script Reference"=w885:T4, "Data Address Endianness"=w883:bool, "WRITE"=w880:u8, "EEPROM Address (u8)"=w875:u16, "Number of Bytes (Read)"=w872:i16, "Target Page Size (bytes)"=w874:i32, "Bit Pattern (Write All)"=w871:T3)
        n345 = for {
          N: w872 -> [_]
          tunnel: w871 -> [w891]
          tunnel: [w890] -> w870 mode=indexing
          n346 = case shown="\"0xAA (0b10101010)\"" w891 {
            tunnel: [u8 255 u8 0 u8 170 u8 85] -> w890
            frame "All ONES", Default {
            }
            frame "All ZEROES" {
            }
            frame "0xAA (0b10101010)" {
            }
            frame "0x55 (0b01010101)" {
            }
          }
        }
        n347 = call "CreateWriteCluster.vi"("Page Size in Bytes"=w874, "EEPROM Starting Address"=w875, "Number of Bytes to Write"=w872) -> ("Array of Write Cluster Information"=w873:T9)  [unwired: 1 in]
        n348 = for {
          tunnel: w887 -> [w905]
          tunnel: w885 -> [w904]
          tunnel: w884 -> [_]
          tunnel: w876 -> [w926]
          tunnel: w883 -> [w925]
          tunnel: [w924] -> w881
          tunnel: w880 -> [w923]
          tunnel: w877 -> [w916]
          tunnel: w878 -> [w915]
          tunnel: [w917] -> w879
          tunnel: w878 -> [w903]
          tunnel: w877 -> [w902]
          tunnel: w873 -> [w901] mode=indexing
          tunnel: w870 -> [w898]
          w907 = 2 ("index")
          # "Tcsl"
          n349 = Select(t=i16 0, s=w925, f=i16 -8) -> (s? t:f=w912:i16)
          n350 = Unbundle By Name(w901) -> ("EEPROM Address"=w900:u16, "Data Index"=w897:u32, "Length"=w899:u32)
          n351 = Rotate(1:w900, 2:w912) -> (0:w909:u16)
          n352 = Array Subset(array=w898, index=w897, length=w899) -> (w896:u8[])
          n353 = case shown="\"8 bits\"" w926 {
            tunnel: [w953 w955] -> w908
            tunnel: w909 -> [w952 w956]
            tunnel: w923 -> [w942 w957]
            tunnel: w925 -> [w950 _]
            tunnel: w896 -> [w938 w954]
            tunnel: w900 -> [w937 _]
            frame "8 bits" {
              n354 = Number To Boolean Array(number=w937) -> (Boolean array=w941:bool[])
              n355 = Split Number(x=w952) -> (hi(x)=w951:u8, lo(x)=w949:u8)
              n356 = Number To Boolean Array(number=w942) -> (Boolean array=w947:bool[])
              n357 = Index Array(array=w941, index=8) -> (element=w939:bool)
              n358 = Replace Array Subset(array=w947, new element=w939, index=3) -> (w945:bool[])
              n359 = Boolean Array To Number(Boolean array=w945) -> (number=w944:u32)
              n360 = Select(t=w949, s=w950, f=w951) -> (s? t:f=w948:u8)
              n361 = To Unsigned Byte Integer(number=w944) -> (unsigned 8bit integer=w943:u8)
              n362 = Build Array (concatenate)(w943, w948, w938) -> (w953:u8[])
            }
            frame "16 bits", Default {
              n363 = Split Number(x=w956) -> (hi(x)=w958:u8, lo(x)=w959:u8)
              n364 = Build Array (concatenate)(w957, w958, w959, w954) -> (w955:u8[])
            }
          }
          n365 = case shown="\"Low (Assert High)\"" w903 {
            tunnel: [w931 w936] -> w911
            tunnel: [w930 w935] -> w910
            tunnel: w905 -> [w929 w934]
            tunnel: w904 -> [w928 w933]
            tunnel: w902 -> [w927 w932]
            frame "High (Assert Low)" {
              n366 = call <vilib>:"NI-845x SPI Script CS Low.vi"("error in (no error)"=w929, "chip select (0)"=w927, "spi script reference in"=w928) -> ("error out"=w930:errorcluster, "spi script reference out"=w931:T4)  [unwired: 7 in]
            }
            frame "Low (Assert High)" {
              n367 = call <vilib>:"NI-845x SPI Script CS High.vi"("error in (no error)"=w934, "chip select (0)"=w932, "spi script reference in"=w933) -> ("error out"=w935:errorcluster, "spi script reference out"=w936:T4)  [unwired: 7 in]
            }
          }
          n368 = call <vilib>:"NI-845x SPI Script Write Read.vi"("error in (no error)"=w910, "write data"=w908, "spi script reference in"=w911) -> ("error out"=w922:errorcluster, "script read index"=w924:u32, "spi script reference out"=w921:T4)  [unwired: 1 in, 5 out]
          n369 = Array Subset(array=w908, index=w907, length=w907) -> (w906:u8[])
          n370 = case shown="\"Low (Assert High)\"" w915 {
            tunnel: [w964 w969] -> w920
            tunnel: [w963 w968] -> w919
            tunnel: w922 -> [w962 w967]
            tunnel: w921 -> [w961 w966]
            tunnel: w916 -> [w960 w965]
            frame "High (Assert Low)" {
              n371 = call <vilib>:"NI-845x SPI Script CS High.vi"("error in (no error)"=w962, "chip select (0)"=w960, "spi script reference in"=w961) -> ("error out"=w964:errorcluster, "spi script reference out"=w963:T4)  [unwired: 7 in]
            }
            frame "Low (Assert High)" {
              n372 = call <vilib>:"NI-845x SPI Script CS Low.vi"("error in (no error)"=w967, "chip select (0)"=w965, "spi script reference in"=w966) -> ("error out"=w969:errorcluster, "spi script reference out"=w968:T4)  [unwired: 7 in]
            }
          }
          n373 = local write "Data Bytes Written"(w906) -> ()
          n374 = call-poly <vilib>:"NI-845x SPI Script Delay.vi"("error in (no error)"=w920, "delay in microseconds (0)"=u16 1, "spi script reference in"=w919) -> ("error out"=w917:errorcluster)  [unwired: 8 out]
        }
        n375 = Bundle By Name(cluster=w886, "script read index"=w881) -> (w882:T7)
        n376 = call <vilib>:"Add State(s) to Queue__JKI_lib_State_Machine.vi"("State(s) in (\"\")"=w889) -> ("States Out"=w888:string)  [unwired: 14 in]
      }
      frame "NI8451: EWDS" {
        w983 = u8 0
        # "1. Send SB & EWDS Opcode\n2. A dummy address byte\n3. A dummy data byte"
        n377 = Unbundle By Name(w978) -> ("EWDS"=w976:u8, "SPI Script Reference"=w972:T4, "CS/SS"=w973:u32, "CS Idle Level"=w974:enum16{"Low (Assert High)", "High (Assert Low)"})
        n378 = case shown="\"High (Assert Low)\"" w974 {
          tunnel: w972 -> [w990 w995]
          tunnel: w975 -> [w989 w994]
          tunnel: [w988 w993] -> _
          tunnel: w973 -> [w987 w992]
          tunnel: [w986 w991] -> w971
          frame "High (Assert Low)" {
            n379 = call <vilib>:"NI-845x SPI Script CS High.vi"("error in (no error)"=w989, "chip select (0)"=w987, "spi script reference in"=w990) -> ("error out"=w988:errorcluster, "spi script reference out"=w986:T4)  [unwired: 7 in]
          }
          frame "Low (Assert High)" {
            n380 = call <vilib>:"NI-845x SPI Script CS Low.vi"("error in (no error)"=w994, "chip select (0)"=w992, "spi script reference in"=w995) -> ("error out"=w993:errorcluster, "spi script reference out"=w991:T4)  [unwired: 7 in]
          }
        }
        n381 = case shown="\"High (Assert Low)\"" w974 {
          tunnel: w975 -> [w1008 w1013]
          tunnel: w971 -> [w1007 w1012]
          tunnel: [w1006 w1011] -> w977
          tunnel: w973 -> [w1005 w1010]
          tunnel: [w1004 w1009] -> w970
          frame "High (Assert Low)" {
            n382 = call <vilib>:"NI-845x SPI Script CS Low.vi"("error in (no error)"=w1008, "chip select (0)"=w1005, "spi script reference in"=w1007) -> ("error out"=w1004:errorcluster, "spi script reference out"=w1006:T4)  [unwired: 7 in]
          }
          frame "Low (Assert High)" {
            n383 = call <vilib>:"NI-845x SPI Script CS High.vi"("error in (no error)"=w1013, "chip select (0)"=w1010, "spi script reference in"=w1012) -> ("error out"=w1009:errorcluster, "spi script reference out"=w1011:T4)  [unwired: 7 in]
          }
        }
        n384 = Build Array(w976, w983, w983) -> (w982:u8[])
        n385 = call <vilib>:"NI-845x SPI Script Write Read.vi"("error in (no error)"=w970, "write data"=w982, "spi script reference in"=w977) -> ("error out"=w980:errorcluster, "spi script reference out"=w981:T4)  [unwired: 1 in, 6 out]
        n386 = case shown="\"Low (Assert High)\"" w974 {
          tunnel: w981 -> [w999 w1003]
          tunnel: w980 -> [w998 w1002]
          tunnel: [w997 w1001] -> w979
          tunnel: w973 -> [w996 w1000]
          frame "High (Assert Low)" {
            n387 = call <vilib>:"NI-845x SPI Script CS High.vi"("error in (no error)"=w998, "chip select (0)"=w996, "spi script reference in"=w999) -> ("error out"=w997:errorcluster)  [unwired: 7 in, 1 out]
          }
          frame "Low (Assert High)" {
            n388 = call <vilib>:"NI-845x SPI Script CS Low.vi"("error in (no error)"=w1002, "chip select (0)"=w1000, "spi script reference in"=w1003) -> ("error out"=w1001:errorcluster)  [unwired: 7 in, 1 out]
          }
        }
        n389 = call <vilib>:"Add State(s) to Queue__JKI_lib_State_Machine.vi"("State(s) in (\"\")"=w985) -> ("States Out"=w984:string)  [unwired: 14 in]
      }
      frame "NI8451: Erase ALL" {
        # "Then assert the CS line\nto start the ERASE ALL\ncycle. The ERASE ALL\ncycle is self-timed. \nNo need to CLK"
        # "Delay for Tcsl"
        # "1. Send SB & ERAL Opcode\n2. A dummy address byte\n3. A dummy data byte"
        n390 = Unbundle By Name(w1033) -> ("EEPROM Device Type"=w1020:enum16{"Microchip 93C86", "Microchip LC56BT"}, "ERAL"=w1030:u8, "SPI Script Reference"=w1032:T4, "CS/SS"=w1023:u32, "CS Idle Level"=w1022:enum16{"Low (Assert High)", "High (Assert Low)"}, "Page Write Delay (ms)"=w1014:u8)
        n391 = case shown="\"Microchip LC56BT\"" w1020 {
          tunnel: [w1043 w1047] -> w1037
          tunnel: w1030 -> [w1042 w1046]
          frame "Microchip LC56BT" {
            w1041 = u8 0 ("element")
            # "16-bit Data & 8-bit Address"
            n392 = To Unsigned Byte Integer(number=w1042) -> (unsigned 8bit integer=w1040:u8)
            n393 = Build Array(w1040, w1041, w1041) -> (w1043:u8[])
          }
          frame "Microchip 93C86" {
            w1044 = u16 0 ("element")
            # "16-bit Data & Address"
            n394 = To Unsigned Word Integer(number=w1046) -> (unsigned 16bit integer=w1045:u16)
            n395 = Build Array(w1045, w1044, w1044) -> (w1047:u16[])
          }
        }
        n396 = case shown="\"Low (Assert High)\"" w1022 {
          tunnel: w1034 -> [w1072 w1077]
          tunnel: w1032 -> [w1071 w1076]
          tunnel: [w1070 w1075] -> w1031
          tunnel: w1023 -> [w1069 w1074]
          tunnel: [w1068 w1073] -> w1026
          frame "High (Assert Low)" {
            n397 = call <vilib>:"NI-845x SPI Script CS Low.vi"("error in (no error)"=w1072, "chip select (0)"=w1069, "spi script reference in"=w1071) -> ("error out"=w1068:errorcluster, "spi script reference out"=w1070:T4)  [unwired: 7 in]
          }
          frame "Low (Assert High)" {
            n398 = call <vilib>:"NI-845x SPI Script CS High.vi"("error in (no error)"=w1077, "chip select (0)"=w1074, "spi script reference in"=w1076) -> ("error out"=w1073:errorcluster, "spi script reference out"=w1075:T4)  [unwired: 7 in]
          }
        }
        n399 = call <vilib>:"NI-845x SPI Script Write Read.vi"("error in (no error)"=w1026, "write data"=w1037, "spi script reference in"=w1031) -> ("error out"=w1035:errorcluster, "script read index"=w1018:u32, "spi script reference out"=w1036:T4)  [unwired: 1 in, 5 out]
        n400 = case shown="\"Low (Assert High)\"" w1022 {
          tunnel: w1036 -> [w1062 w1067]
          tunnel: w1035 -> [w1061 w1066]
          tunnel: [w1060 w1065] -> w1029
          tunnel: w1023 -> [w1059 w1064]
          tunnel: [w1058 w1063] -> w1028
          frame "High (Assert Low)" {
            n401 = call <vilib>:"NI-845x SPI Script CS High.vi"("error in (no error)"=w1061, "chip select (0)"=w1059, "spi script reference in"=w1062) -> ("error out"=w1060:errorcluster, "spi script reference out"=w1058:T4)  [unwired: 7 in]
          }
          frame "Low (Assert High)" {
            n402 = call <vilib>:"NI-845x SPI Script CS Low.vi"("error in (no error)"=w1066, "chip select (0)"=w1064, "spi script reference in"=w1067) -> ("error out"=w1065:errorcluster, "spi script reference out"=w1063:T4)  [unwired: 7 in]
          }
        }
        n403 = Bundle By Name(cluster=w1033, "script read index"=w1018) -> (w1019:T7)
        n404 = call-poly <vilib>:"NI-845x SPI Script Delay.vi"("error in (no error)"=w1029, "delay in microseconds (0)"=u16 1, "spi script reference in"=w1028) -> ("error out"=w1025:errorcluster, "spi script reference out"=w1024:T4)  [unwired: 7 in]
        n405 = case shown="\"Low (Assert High)\"" w1022 {
          tunnel: w1025 -> [w1052 w1057]
          tunnel: w1024 -> [w1049 w1056]
          tunnel: w1023 -> [w1051 w1055]
          tunnel: [w1050 w1054] -> w1017
          tunnel: [w1048 w1053] -> w1016
          frame "High (Assert Low)" {
            n406 = call <vilib>:"NI-845x SPI Script CS Low.vi"("error in (no error)"=w1052, "chip select (0)"=w1051, "spi script reference in"=w1049) -> ("error out"=w1050:errorcluster, "spi script reference out"=w1048:T4)  [unwired: 7 in]
          }
          frame "Low (Assert High)" {
            n407 = call <vilib>:"NI-845x SPI Script CS High.vi"("error in (no error)"=w1057, "chip select (0)"=w1055, "spi script reference in"=w1056) -> ("error out"=w1054:errorcluster, "spi script reference out"=w1053:T4)  [unwired: 7 in]
          }
        }
        n408 = call <vilib>:"Add State(s) to Queue__JKI_lib_State_Machine.vi"("State(s) in Front (\"\")"="UI: Display Message >>  [Alert!][ERASE ALL Completed][10000]" ("State(s) in Front (\"\")"), "State(s) in (\"\")"=w1039) -> ("States Out"=w1038:string)  [unwired: 13 in]
        n409 = call-poly <vilib>:"NI-845x SPI Script Delay.vi"("error in (no error)"=w1017, "delay in milliseconds (0)"=w1014, "spi script reference in"=w1016) -> ("error out"=w1015:errorcluster)  [unwired: 7 in, 1 out]
      }
      frame "NI8451: Write ALL" {
        # "Then assert the CS line\nto start the ERASE ALL\ncycle. The ERASE ALL\ncycle is self-timed. \nNo need to CLK"
        # "Delay for Tcsl"
        # "1. Send SB & WRAL opcode.\n2. A dummy address byte.\n3. Desired data pattern to write."
        n410 = Unbundle By Name(w1098) -> ("WRAL"=w1096:u8, "EEPROM Device Type"=w1087:enum16{"Microchip 93C86", "Microchip LC56BT"}, "Bit Pattern (Write All)"=w1089:T3, "SPI Script Reference"=w1078:T4, "CS/SS"=w1080:u32, "Page Write Delay (ms)"=w1081:u8)  [unwired: 1 out]
        n411 = case shown="\"Microchip LC56BT\"" w1087 {
          tunnel: [w1109 w1119] -> w1101
          tunnel: w1096 -> [w1108 w1118]
          tunnel: w1089 -> [w1107 w1117]
          frame "Microchip LC56BT" {
            # "16-bit Data & 8-bit Address"
            n412 = case shown="\"0xEE (0b11101110)\"" w1107 {
              tunnel: [u8 255 u8 0 u8 238 u8 170 u8 85] -> w1106
              frame "All ONES", Default {
              }
              frame "All ZEROES" {
              }
              frame "0xEE (0b11101110)" {
              }
              frame "0xAA (0b10101010)" {
              }
              frame "0x55 (0b01010101)" {
              }
            }
            n413 = To Unsigned Byte Integer(number=w1108) -> (unsigned 8bit integer=w1105:u8)
            n414 = Build Array(w1105, u8 0 ("element"), w1106, w1106) -> (w1109:u8[])
          }
          frame "Microchip 93C86", Default {
            # "16-bit Data & Address"
            n415 = case shown="\"0x55 (0b01010101)\"" w1117 {
              tunnel: [u16 65535 u16 0 u16 61166 u16 43690 u16 21845] -> w1115
              frame "All ONES", Default {
              }
              frame "All ZEROES" {
              }
              frame "0xEE (0b11101110)" {
              }
              frame "0xAA (0b10101010)" {
              }
              frame "0x55 (0b01010101)" {
              }
            }
            n416 = To Unsigned Word Integer(number=w1118) -> (unsigned 16bit integer=w1116:u16)
            n417 = Build Array(w1116, w1115, w1115, w1115) -> (w1119:u16[])
          }
        }
        n418 = call <vilib>:"NI-845x SPI Script CS High.vi"("error in (no error)"=w1079, "chip select (0)"=w1080, "spi script reference in"=w1078) -> ("error out"=w1092:errorcluster, "spi script reference out"=w1097:T4)  [unwired: 7 in]
        n419 = call <vilib>:"NI-845x SPI Script Write Read.vi"("error in (no error)"=w1092, "write data"=w1101, "spi script reference in"=w1097) -> ("error out"=w1099:errorcluster, "script read index"=w1085:u32, "spi script reference out"=w1100:T4)  [unwired: 1 in, 5 out]
        n420 = Bundle By Name(cluster=w1098, "script read index"=w1085) -> (w1086:T7)
        n421 = call <vilib>:"NI-845x SPI Script CS Low.vi"("error in (no error)"=w1099, "chip select (0)"=w1080, "spi script reference in"=w1100) -> ("error out"=w1095:errorcluster, "spi script reference out"=w1094:T4)  [unwired: 7 in]
        n422 = call-poly <vilib>:"NI-845x SPI Script Delay.vi"("error in (no error)"=w1095, "delay in microseconds (0)"=u16 2, "spi script reference in"=w1094) -> ("error out"=w1091:errorcluster, "spi script reference out"=w1090:T4)  [unwired: 7 in]
        n423 = call <vilib>:"NI-845x SPI Script CS High.vi"("error in (no error)"=w1091, "chip select (0)"=w1080, "spi script reference in"=w1090) -> ("error out"=w1083:errorcluster, "spi script reference out"=w1084:T4)  [unwired: 7 in]
        n424 = call <vilib>:"Add State(s) to Queue__JKI_lib_State_Machine.vi"("State(s) in Front (\"\")"="UI: Display Message >>  [Alert!][WRITE ALL Completed][10000]" ("State(s) in Front (\"\")"), "State(s) in (\"\")"=w1103) -> ("States Out"=w1102:string)  [unwired: 13 in]
        n425 = call-poly <vilib>:"NI-845x SPI Script Delay.vi"("error in (no error)"=w1083, "delay in milliseconds (0)"=w1081, "spi script reference in"=w1084) -> ("error out"=w1082:errorcluster)  [unwired: 7 in, 1 out]
      }
      frame "NI8451: RUN Script - Read Data - Close Device" {
        # "Close SPI bus, Run Script, Read the Data Array from Device, Close the reference to Device"
        n426 = Unbundle By Name(w1136) -> ("EEPROM Device Type"=w1127:enum16{"Microchip 93C86", "Microchip LC56BT"}, "script read index"=w1130:u32, "NI8451 Device ID"=w1129:T2, "SPI Script Reference"=w1137:T4)
        n427 = case shown="\"Microchip LC56BT\"" w1127 {
          tunnel: [3 ("index") 2 ("index")] -> w1128
          frame "Microchip 93C86", Default {
          }
          frame "Microchip LC56BT" {
          }
        }
        n428 = call <vilib>:"NI-845x SPI Script Disable SPI.vi"("error in (no error)"=w1139, "spi script reference in"=w1137) -> ("error out"=w1140:errorcluster, "spi script reference out"=w1141:T4)  [unwired: 8 out]
        n429 = call <vilib>:"NI-845x SPI Run Script.vi"("error in (no error)"=w1140, "device reference in"=w1129, "spi script reference in"=w1141) -> ("error out"=w1134:errorcluster, "spi script reference out"=w1135:T4)  [unwired: 1 in, 6 out]
        n430 = call <vilib>:"NI-845x SPI Extract Script Read Data.vi"("error in (no error)"=w1134, "script read index"=w1130, "spi script reference in"=w1135) -> ("error out"=w1133:errorcluster, "read data"=w1131:u8[], "spi script reference out"=w1132:T4)  [unwired: 6 out]
        n431 = Array Subset(array=w1131, index=w1128) -> (w1125:u8[])  [unwired: 1 in]
        n432 = call-poly <vilib>:"NI-845x Close Reference.vi"("error in (no error)"=w1133, "spi script reference"=w1132) -> ("error out"=w1138:errorcluster)  [unwired: 9 out]
        n433 = local write "Read Data"(w1125) -> ()
        n434 = Bundle By Name(cluster=w1136, "Read Data"=w1125) -> (w1126:T7)
        n435 = call <vilib>:"Add State(s) to Queue__JKI_lib_State_Machine.vi"("State(s) in (\"\")"=w1143) -> ("States Out"=w1142:string)  [unwired: 14 in]
      }
      frame "NI8451: Run Script - Close SPI - Close Device" {
        n436 = Unbundle By Name(w1149) -> ("NI8451 Device ID"=w1146:T2, "SPI Script Reference"=w1150:T4)
        n437 = call <vilib>:"NI-845x SPI Script Disable SPI.vi"("error in (no error)"=w1152, "spi script reference in"=w1150) -> ("error out"=w1153:errorcluster, "spi script reference out"=w1154:T4)  [unwired: 8 out]
        n438 = call <vilib>:"NI-845x SPI Run Script.vi"("error in (no error)"=w1153, "device reference in"=w1146, "spi script reference in"=w1154) -> ("error out"=w1147:errorcluster, "spi script reference out"=w1148:T4)  [unwired: 1 in, 6 out]
        n439 = call-poly <vilib>:"NI-845x Close Reference.vi"("error in (no error)"=w1147, "spi script reference"=w1148) -> ("error out"=w1151:errorcluster)  [unwired: 9 out]
        n440 = call <vilib>:"Add State(s) to Queue__JKI_lib_State_Machine.vi"("State(s) in (\"\")"=w1156) -> ("States Out"=w1155:string)  [unwired: 14 in]
      }
    }
  }
